vi "Batch_main_with_graph.vi"(1 "Stop":bool=TRUE, 2 "ExpFilePath":path=path "C:/Documents and Settings/Bauerle/Mes documents/takada/HBT6/201612181913.h5") -> ()   [LabVIEW 2013]
uses:
  <vilib>/addons/h5labview2/base/hid_t.ctl
  fpga-bitfile-ref.ctl
  host-subvis/Fast_sequence/sequence slot/slot-use.ctl
  host-subvis/Fast_sequence/sequence slot/triggers.ctl
  host-subvis/Fast_sequence/sequence slot/DAC.ctl
  host-subvis/Fast_sequence/sequence slot/DAC_fastseq-offset.ctl
  host-subvis/Fast_sequence/sequence slot/timing.ctl
  host-subvis/Fast_sequence/sequence slot/jump.ctl
  <vilib>/addons/h5labview2/file/H5Fmode.ctl
  <vilib>/addons/h5labview2/base/lib_path.vi
  <vilib>/addons/h5labview2/base/H5Equery.vi
  <vilib>/FPGAPlugInAG/sbRIO-9602/niLvFpga_Close_sbRIO-9602.vi
  <vilib>/addons/h5labview2/dataset/H5Dread.llb/H5Dread.xnode
  <vilib>/addons/h5labview2/attrib/H5Aread.llb/H5Aread.xnode
  <vilib>/rvi/interface/nirviCloseFPGA/nirviCloseFPGA.xnode
  FPGA Bitfiles/fpga-clean1_FPGATarget_FPGAMAINlock-in_FC21E42C.lvbitx
  <vilib>/addons/h5labview2/attrib/H5Awrite.llb/H5Awrite.xnode
  <vilib>/addons/h5labview2/file/H5F.lvlib
  <vilib>/addons/h5labview2/dataset/H5D.lvlib
  <vilib>/addons/h5labview2/space/H5S.lvlib
panel:
  out "Remaning time (min)":dbl
  in  "temp file interval (ms)":i32=600
  in  "get variable interval (ms)":i32=300
  out "Graph":T1(graph)
  in  "Plot parameters":T2
  out "Temp data":sgl[][](array[numeric])
  out "Initial positions":T3(array[cluster])=[{"Name"="AWG", "kind"=7, "Value"=0.0}, {"Name"="Freq", "kind"=6, "Value"=2759965000.0}, {"Name"="Power", "kind"=6, "Value"=-40.0}, {"Name"="sus", "kind"=4, "Value"=0.29998779296875}, {"Name"="rus", "kind"=4, "Value"=0.29998779296875}, {"Name"="rls", "kind"=4, "Value"=0.29998779296875}, {"Name"="sls", "kind"=4, "Value"=0.059967041015625}, {"Name"="suq", "kind"=4, "Value"=-1.75994873046875}, {"Name"="suu", "kind"=4, "Value"=-0.749969482421875}, {"Name"="sur", "kind"=4, "Value"=-1.199951171875}, {"Name"="suc", "kind"=4, "Value"=-0.449981689453125}, {"Name"="sul", "kind"=4, "Value"=-0.89996337890625}, {"Name"="ruq", "kind"=4, "Value"=-1.699981689453125}, {"Name"="ruu", "kind"=4, "Value"=-0.749969482421875}, {"Name"="rur", "kind"=4, "Value"=-1.25}, {"Name"="ruc", "kind"=4, "Value"=-0.399932861328125}, {"Name"="rul", "kind"=4, "Value"=-0.89996337890625}, {"Name"="rlq", "kind"=4, "Value"=-1.7999267578125}, {"Name"="rlu", "kind"=4, "Value"=-0.89996337890625}, {"Name"="rlr", "kind"=4, "Value"=-1.199951171875}, {"Name"="rlc", "kind"=4, "Value"=-0.5999755859375}, {"Name"="rll", "kind"=4, "Value"=-0.749969482421875}, {"Name"="slq", "kind"=4, "Value"=-1.62506103515625}, {"Name"="slu", "kind"=4, "Value"=-0.89996337890625}, {"Name"="slr", "kind"=4, "Value"=-1.150054931640625}, {"Name"="slc", "kind"=4, "Value"=-0.449981689453125}, {"Name"="sll", "kind"=4, "Value"=-0.749969482421875}, {"Name"="tu", "kind"=4, "Value"=-0.89996337890625}, {"Name"="t", "kind"=4, "Value"=-0.89996337890625}, {"Name"="tl", "kind"=4, "Value"=-0.89996337890625}, {"Name"="4:7", "kind"=4, "Value"=-1.00006103515625}]
  in  "Buf size":i32=300
  out "Var index":u64[](array[numeric])=[0, 49, 0]
  out "start read vals":bool=TRUE
  out "Indexes File":u64[](array[numeric])=[8, 21, 0]
  out "Finish":bool=TRUE
  out "error out":errorcluster
  in  "File update interval (sec)":i32=3000000
  out "DAC_lock-in_info":T4={"Kind"=5, "Strings"=["DAC_Lock-in", "10.0.0.2", "V"], "uint64s"=[0, 1, 0, 0], "Doubles"=[1.0, 0.0, -1.0, -1.0, 50.0, 0.10000000149011612], "DAQmx take out list"=[]}
  out "Fast sequence parameters":T11={"Sequence size"=22, "IP address"="10.0.0.2", "Fast-seq-divider"=6661, "Trigger length"=300, "Sample count"=100, "Send all points?"=FALSE, "Upper limit"=1.0, "Lower limit"=-1.0, "Start ramp at"=0, "fast channels"=[{"dummy?"=FALSE, "panel"=0, "channel"=7}, {"dummy?"=FALSE, "panel"=1, "channel"=0}, {"dummy?"=FALSE, "panel"=0, "channel"=5}, {"dummy?"=FALSE, "panel"=1, "channel"=5}, {"dummy?"=FALSE, "panel"=1, "channel"=6}, {"dummy?"=FALSE, "panel"=1, "channel"=2}, {"dummy?"=FALSE, "panel"=2, "channel"=2}, {"dummy?"=FALSE, "panel"=2, "channel"=3}, {"dummy?"=FALSE, "panel"=2, "channel"=0}, {"dummy?"=FALSE, "panel"=2, "channel"=7}, {"dummy?"=FALSE, "panel"=3, "channel"=0}, {"dummy?"=FALSE, "panel"=2, "channel"=5}, {"dummy?"=FALSE, "panel"=3, "channel"=2}, {"dummy?"=FALSE, "panel"=3, "channel"=3}, {"dummy?"=FALSE, "panel"=3, "channel"=4}, {"dummy?"=FALSE, "panel"=4, "channel"=7}], "fastseq"=[{"use"=enum."triggers", "Triggers"={"triggers"={"1"=TRUE, "2"=TRUE, "3"=FALSE, "4"=FALSE}, "stop"=FALSE}, "DAC"={"FastChanNum"=0, "DAC offset"=0.0}, "timing"=0.0, "slot#"=0}, {"use"=enum."timing", "Triggers"={"triggers"={"1"=FALSE, "2"=FALSE, "3"=FALSE, "4"=FALSE}, "stop"=FALSE}, "DAC"={"FastChanNum"=0, "DAC offset"=0.0}, "timing"=1.0, "slot#"=0}, {"use"=enum."triggers", "Triggers"={"triggers"={"1"=TRUE, "2"=FALSE, "3"=FALSE, "4"=FALSE}, "stop"=FALSE}, "DAC"={"FastChanNum"=0, "DAC offset"=0.0}, "timing"=0.0, "slot#"=0}, {"use"=enum."timing", "Triggers"={"triggers"={"1"=FALSE, "2"=FALSE, "3"=FALSE, "4"=FALSE}, "stop"=FALSE}, "DAC"={"FastChanNum"=0, "DAC offset"=0.0}, "timing"=1.0, "slot#"=0}, {"use"=enum."DAC", "Triggers"={"triggers"={"1"=FALSE, "2"=FALSE, "3"=FALSE, "4"=FALSE}, "stop"=FALSE}, "DAC"={"FastChanNum"=1, "DAC offset"=0.0}, "timing"=0.0, "slot#"=0}, {"use"=enum."DAC", "Triggers"={"triggers"={"1"=FALSE, "2"=FALSE, "3"=FALSE, "4"=FALSE}, "stop"=FALSE}, "DAC"={"FastChanNum"=0, "DAC offset"=0.0}, "timing"=0.0, "slot#"=0}, {"use"=enum."DAC", "Triggers"={"triggers"={"1"=FALSE, "2"=FALSE, "3"=FALSE, "4"=FALSE}, "stop"=FALSE}, "DAC"={"FastChanNum"=4, "DAC offset"=0.0}, "timing"=0.0, "slot#"=0}, {"use"=enum."DAC", "Triggers"={"triggers"={"1"=FALSE, "2"=FALSE, "3"=FALSE, "4"=FALSE}, "stop"=FALSE}, "DAC"={"FastChanNum"=3, "DAC offset"=0.0}, "timing"=0.0, "slot#"=0}, {"use"=enum."DAC", "Triggers"={"triggers"={"1"=FALSE, "2"=FALSE, "3"=FALSE, "4"=FALSE}, "stop"=FALSE}, "DAC"={"FastChanNum"=7, "DAC offset"=0.0}, "timing"=0.0, "slot#"=0}, {"use"=enum."DAC", "Triggers"={"triggers"={"1"=FALSE, "2"=FALSE, "3"=FALSE, "4"=FALSE}, "stop"=FALSE}, "DAC"={"FastChanNum"=6, "DAC offset"=0.0}, "timing"=0.0, "slot#"=0}, {"use"=enum."DAC", "Triggers"={"triggers"={"1"=FALSE, "2"=FALSE, "3"=FALSE, "4"=FALSE}, "stop"=FALSE}, "DAC"={"FastChanNum"=10, "DAC offset"=0.0}, "timing"=0.0, "slot#"=0}, {"use"=enum."DAC", "Triggers"={"triggers"={"1"=FALSE, "2"=FALSE, "3"=FALSE, "4"=FALSE}, "stop"=FALSE}, "DAC"={"FastChanNum"=9, "DAC offset"=0.0}, "timing"=0.0, "slot#"=0}, {"use"=enum."timing", "Triggers"={"triggers"={"1"=FALSE, "2"=FALSE, "3"=FALSE, "4"=FALSE}, "stop"=FALSE}, "DAC"={"FastChanNum"=0, "DAC offset"=0.0}, "timing"=10.0, "slot#"=0}, {"use"=enum."DAC", "Triggers"={"triggers"={"1"=FALSE, "2"=FALSE, "3"=FALSE, "4"=FALSE}, "stop"=FALSE}, "DAC"={"FastChanNum"=1, "DAC offset"=0.0}, "timing"=0.0, "slot#"=0}, {"use"=enum."DAC", "Triggers"={"triggers"={"1"=FALSE, "2"=FALSE, "3"=FALSE, "4"=FALSE}, "stop"=FALSE}, "DAC"={"FastChanNum"=0, "DAC offset"=0.0}, "timing"=0.0, "slot#"=0}, {"use"=enum."DAC", "Triggers"={"triggers"={"1"=FALSE, "2"=FALSE, "3"=FALSE, "4"=FALSE}, "stop"=FALSE}, "DAC"={"FastChanNum"=4, "DAC offset"=0.0}, "timing"=0.0, "slot#"=0}, {"use"=enum."DAC", "Triggers"={"triggers"={"1"=FALSE, "2"=FALSE, "3"=FALSE, "4"=FALSE}, "stop"=FALSE}, "DAC"={"FastChanNum"=3, "DAC offset"=0.0}, "timing"=0.0, "slot#"=0}, {"use"=enum."DAC", "Triggers"={"triggers"={"1"=FALSE, "2"=FALSE, "3"=FALSE, "4"=FALSE}, "stop"=FALSE}, "DAC"={"FastChanNum"=7, "DAC offset"=0.0}, "timing"=0.0, "slot#"=0}, {"use"=enum."DAC", "Triggers"={"triggers"={"1"=FALSE, "2"=FALSE, "3"=FALSE, "4"=FALSE}, "stop"=FALSE}, "DAC"={"FastChanNum"=6, "DAC offset"=0.0}, "timing"=0.0, "slot#"=0}, {"use"=enum."DAC", "Triggers"={"triggers"={"1"=FALSE, "2"=FALSE, "3"=FALSE, "4"=FALSE}, "stop"=FALSE}, "DAC"={"FastChanNum"=10, "DAC offset"=0.0}, "timing"=0.0, "slot#"=0}, {"use"=enum."DAC", "Triggers"={"triggers"={"1"=FALSE, "2"=FALSE, "3"=FALSE, "4"=FALSE}, "stop"=FALSE}, "DAC"={"FastChanNum"=9, "DAC offset"=0.0}, "timing"=0.0, "slot#"=0}, {"use"=enum."jump", "Triggers"={"triggers"={"1"=FALSE, "2"=FALSE, "3"=FALSE, "4"=FALSE}, "stop"=FALSE}, "DAC"={"FastChanNum"=0, "DAC offset"=0.0}, "timing"=0.0, "slot#"=21}]} {"fastseq"."DAC"."DAC offset" min=-1 max=0.5; "fastseq"."DAC"."FastChanNum" max=15 step=1; "fastseq"."slot#" max=4095}
  out "Timings":dbl[][](array[numeric])=[[2417234066.0, 52858.0]] format="%^_3e"
  out "Indexes":i32[](array[numeric])=[8, 21, 0]
  out "sweep_dim":u64[](array[numeric])=[11, 61, 61]
  out "Readout parameters":T12(array[cluster])=[{"Kind"=0, "Strings"=["ADC", "", "V", "sud;rud;rld;sld", "nA;nA;nA;nA", "100.0;100.0;100.0;100.0"], "uint64s"=[5, 4, 250000, 1, 100, 10106, 1000000, 10000, 0, 1], "Doubles"=[1.0], "DAQmx take out list"=["", ""]}]
  out "Exp_params":T15={"filename"="201612181913", "ExpFilePath"=path "C:/Documents and Settings/Bauerle/Mes documents/takada/HBT6/201612181913.h5", "File Ref list"=[16777217, 33554433, 16777216, 33554432], "sweep_dim"=[11, 61, 61], "sweep_list"=["suq", "ruq", "rlq", "slq", "sur", "rur", "rlr", "slr", "suc", "ruc", "rlc", "slc"], "readout_list"=["sud", "rud", "rld", "sld"], "Sweep instrument bools"=[[0, 0], [0, 0], [0, 0], [0, 0], [0, 0], [0, 0], [0, 0], [0, 0], [0, 0], [0, 0], [0, 0], [0, 0], [0, 0], [0, 0], [0, 0], [0, 0], [0, 0], [0, 0], [0, 0], [0, 0], [0, 0], [0, 0], [0, 0], [0, 0], [0, 0], [0, 0], [0, 0], [0, 0], [0, 0], [0, 0], [0, 0], [0, 0], [0, 0], [0, 0], [0, 0], [0, 0], [0, 0], [0, 0], [0, 0], [0, 0], [0, 0]], "Read out instrument bools"=[[1, 0]], "Experimental bool list"=[TRUE, TRUE], "Initial move"=[{"Name"="None", "kind"=100, "Value"=0.0}], "FPGA Ref"=refnum, "Inst_parameters"={"ConfigFilePath"=path "\\\\10.0.0.7\\takada2/DATA/HBT6/data/Configs/conf_20161218_fc_load.h5", "Inst_list"=["ADC", "AWG", "Freq", "Power", "sus", "rus", "rls", "sls", "suq", "suu", "sur", "suc", "sul", "ruq", "ruu", "rur", "ruc", "rul", "rlq", "rlu", "rlr", "rlc", "rll", "slq", "slu", "slr", "slc", "sll", "tu", "t", "tl", "fast_sequence", "4:7", "suc_load", "sur_load", "ruc_load", "rur_load", "rlc_load", "rlr_load", "slc_load", "slr_load", "load_time"], "fast_mode"=[1, 0], "Wait_times"=[1, 1, 1, 1], "Inst_array"=[{"Kind"=0, "Strings"=["ADC", "", "V", "sud;rud;rld;sld", "nA;nA;nA;nA", "100.0;100.0;100.0;100.0"], "uint64s"=[5, 4, 250000, 1, 100, 10106, 1000000, 1, 0, 1], "Doubles"=[1.0], "DAQmx take out list"=[]}, {"Kind"=7, "Strings"=["AWG", "10.0.0.4", "", "C:\\Documents and Settings\\Bauerle\\Mes documents\\Bautze\\FPGA-clean_works_1.13.6_batchtest\\Python\\AWG", "dummy", "SAWnstrig_v4.py"], "uint64s"=[2, 0, 0, 3, 0, 0, 0, 0, 0, 0, 0, 0, 0, 0], "Doubles"=[1200000000.0, 1.0, 0.0, 1.0, 0.0, 1.0, 0.0, 1.0, 0.0, 1.0, 0.0, 1.0, 0.0], "DAQmx take out list"=[]}, {"Kind"=6, "Strings"=["Freq", "0:19", "GHz"], "uint64s"=[1, 0, 0, 0, 2, 0, 0, 0], "Doubles"=[2.0, -30.0, 200.0, 100.0, 0.0, 6.000999927520752, 9.000000318337698e-06, 30.0, -145.0], "DAQmx take out list"=[]}, {"Kind"=6, "Strings"=["Power", "0:19", "GHz"], "uint64s"=[1, 0, 1, 0, 2, 0, 0, 1], "Doubles"=[2.0, -30.0, 200.0, 100.0, 0.0, 6.000999927520752, 9.000000318337698e-06, 30.0, -145.0], "DAQmx take out list"=[]}, {"Kind"=4, "Strings"=["sus", "10.0.0.2", "mV"], "uint64s"=[0, 1], "Doubles"=[1.0, -1.0, 1.0, -1.0, 1.0], "DAQmx take out list"=[]}, {"Kind"=4, "Strings"=["rus", "10.0.0.2", "mV"], "uint64s"=[0, 2], "Doubles"=[1.0, -1.0, 1.0, -1.0, 1.0], "DAQmx take out list"=[]}, {"Kind"=4, "Strings"=["rls", "10.0.0.2", "mV"], "uint64s"=[0, 3], "Doubles"=[1.0, -1.0, 1.0, -1.0, 1.0], "DAQmx take out list"=[]}, {"Kind"=4, "Strings"=["sls", "10.0.0.2", "mV"], "uint64s"=[0, 4], "Doubles"=[1.0, -1.0, 1.0, -1.0, 1.0], "DAQmx take out list"=[]}, {"Kind"=4, "Strings"=["suq", "10.0.0.2", "V"], "uint64s"=[0, 5], "Doubles"=[0.30000001192092896, -2.0, 1.0, -1.0, 1.0], "DAQmx take out list"=[]}, {"Kind"=4, "Strings"=["suu", "10.0.0.2", "V"], "uint64s"=[0, 6], "Doubles"=[0.30000001192092896, -2.0, 1.0, -1.0, 1.0], "DAQmx take out list"=[]}, {"Kind"=4, "Strings"=["sur", "10.0.0.2", "V"], "uint64s"=[0, 7], "Doubles"=[0.30000001192092896, -2.0, 1.0, -1.0, 1.0], "DAQmx take out list"=[]}, {"Kind"=4, "Strings"=["suc", "10.0.0.2", "V"], "uint64s"=[1, 0], "Doubles"=[0.30000001192092896, -2.0, 1.0, -1.0, 1.0], "DAQmx take out list"=[]}, {"Kind"=4, "Strings"=["sul", "10.0.0.2", "V"], "uint64s"=[1, 1], "Doubles"=[0.30000001192092896, -2.0, 1.0, -1.0, 1.0], "DAQmx take out list"=[]}, {"Kind"=4, "Strings"=["ruq", "10.0.0.2", "V"], "uint64s"=[1, 2], "Doubles"=[0.30000001192092896, -2.0, 1.0, -1.0, 1.0], "DAQmx take out list"=[]}, {"Kind"=4, "Strings"=["ruu", "10.0.0.2", "V"], "uint64s"=[1, 3], "Doubles"=[0.30000001192092896, -2.0, 1.0, -1.0, 1.0], "DAQmx take out list"=[]}, {"Kind"=4, "Strings"=["rur", "10.0.0.2", "V"], "uint64s"=[1, 5], "Doubles"=[0.30000001192092896, -2.0, 1.0, -1.0, 1.0], "DAQmx take out list"=[]}, {"Kind"=4, "Strings"=["ruc", "10.0.0.2", "V"], "uint64s"=[1, 6], "Doubles"=[0.30000001192092896, -2.0, 1.0, -1.0, 1.0], "DAQmx take out list"=[]}, {"Kind"=4, "Strings"=["rul", "10.0.0.2", "V"], "uint64s"=[1, 7], "Doubles"=[0.30000001192092896, -2.0, 1.0, -1.0, 1.0], "DAQmx take out list"=[]}, {"Kind"=4, "Strings"=["rlq", "10.0.0.2", "V"], "uint64s"=[2, 0], "Doubles"=[0.30000001192092896, -2.0, 1.0, -1.0, 1.0], "DAQmx take out list"=[]}, {"Kind"=4, "Strings"=["rlu", "10.0.0.2", "V"], "uint64s"=[2, 1], "Doubles"=[0.30000001192092896, -2.0, 1.0, -1.0, 1.0], "DAQmx take out list"=[]}, {"Kind"=4, "Strings"=["rlr", "10.0.0.2", "V"], "uint64s"=[2, 2], "Doubles"=[0.30000001192092896, -2.0, 1.0, -1.0, 1.0], "DAQmx take out list"=[]}, {"Kind"=4, "Strings"=["rlc", "10.0.0.2", "V"], "uint64s"=[2, 3], "Doubles"=[0.30000001192092896, -2.0, 1.0, -1.0, 1.0], "DAQmx take out list"=[]}, {"Kind"=4, "Strings"=["rll", "10.0.0.2", "V"], "uint64s"=[2, 4], "Doubles"=[0.30000001192092896, -2.0, 1.0, -1.0, 1.0], "DAQmx take out list"=[]}, {"Kind"=4, "Strings"=["slq", "10.0.0.2", "V"], "uint64s"=[2, 5], "Doubles"=[0.30000001192092896, -2.0, 1.0, -1.0, 1.0], "DAQmx take out list"=[]}, {"Kind"=4, "Strings"=["slu", "10.0.0.2", "V"], "uint64s"=[2, 6], "Doubles"=[0.30000001192092896, -2.0, 1.0, -1.0, 1.0], "DAQmx take out list"=[]}, {"Kind"=4, "Strings"=["slr", "10.0.0.2", "V"], "uint64s"=[2, 7], "Doubles"=[0.30000001192092896, -2.0, 1.0, -1.0, 1.0], "DAQmx take out list"=[]}, {"Kind"=4, "Strings"=["slc", "10.0.0.2", "V"], "uint64s"=[3, 0], "Doubles"=[0.30000001192092896, -2.0, 1.0, -1.0, 1.0], "DAQmx take out list"=[]}, {"Kind"=4, "Strings"=["sll", "10.0.0.2", "V"], "uint64s"=[3, 1], "Doubles"=[0.30000001192092896, -2.0, 1.0, -1.0, 1.0], "DAQmx take out list"=[]}, {"Kind"=4, "Strings"=["tu", "10.0.0.2", "V"], "uint64s"=[3, 2], "Doubles"=[0.30000001192092896, -2.0, 1.0, -1.0, 1.0], "DAQmx take out list"=[]}, {"Kind"=4, "Strings"=["t", "10.0.0.2", "V"], "uint64s"=[3, 3], "Doubles"=[0.30000001192092896, -2.0, 1.0, -1.0, 1.0], "DAQmx take out list"=[]}, {"Kind"=4, "Strings"=["tl", "10.0.0.2", "V"], "uint64s"=[3, 4], "Doubles"=[0.30000001192092896, -2.0, 1.0, -1.0, 1.0], "DAQmx take out list"=[]}, {"Kind"=9, "Strings"=["fast_sequence", "10.0.0.2", "V"], "uint64s"=[6661, 300, 100, 0, 7, 8, 5, 13, 14, 10, 18, 19, 16, 23, 24, 21, 26, 27, 28, 39, 0], "Doubles"=[1.0, -1.0, -1.0, -1.0], "DAQmx take out list"=[]}, {"Kind"=4, "Strings"=["4:7", "10.0.0.2", "V"], "uint64s"=[4, 7], "Doubles"=[0.30000001192092896, -2.0, 1.0, -1.0, 1.0], "DAQmx take out list"=[]}, {"Kind"=10, "Strings"=["suc_load", "10.0.0.2", "V"], "uint64s"=[4, 0], "Doubles"=[0.5, -0.5], "DAQmx take out list"=[]}, {"Kind"=10, "Strings"=["sur_load", "10.0.0.2", "V"], "uint64s"=[5, 0], "Doubles"=[0.5, -0.5], "DAQmx take out list"=[]}, {"Kind"=10, "Strings"=["ruc_load", "10.0.0.2", "V"], "uint64s"=[6, 0], "Doubles"=[0.5, -0.5], "DAQmx take out list"=[]}, {"Kind"=10, "Strings"=["rur_load", "10.0.0.2", "V"], "uint64s"=[7, 0], "Doubles"=[0.5, -0.5], "DAQmx take out list"=[]}, {"Kind"=10, "Strings"=["rlc_load", "10.0.0.2", "V"], "uint64s"=[8, 0], "Doubles"=[0.5, -0.5], "DAQmx take out list"=[]}, {"Kind"=10, "Strings"=["rlr_load", "10.0.0.2", "V"], "uint64s"=[9, 0], "Doubles"=[0.5, -0.5], "DAQmx take out list"=[]}, {"Kind"=10, "Strings"=["slc_load", "10.0.0.2", "V"], "uint64s"=[10, 0], "Doubles"=[0.5, -0.5], "DAQmx take out list"=[]}, {"Kind"=10, "Strings"=["slr_load", "10.0.0.2", "V"], "uint64s"=[11, 0], "Doubles"=[0.5, -0.5], "DAQmx take out list"=[]}, {"Kind"=10, "Strings"=["load_time", "10.0.0.2", "ms"], "uint64s"=[12, 0], "Doubles"=[1000.0, -0.009999999776482582], "DAQmx take out list"=[]}]}} {"File Ref list" format="%.0x"}
  out "Sweep inst info":T12(array[cluster])=[{"Kind"=4, "Strings"=["suq", "10.0.0.2", "V"], "uint64s"=[0, 5], "Doubles"=[0.30000001192092896, -2.0, 1.0, -1.0, 1.0], "DAQmx take out list"=[]}, {"Kind"=4, "Strings"=["ruq", "10.0.0.2", "V"], "uint64s"=[1, 2], "Doubles"=[0.30000001192092896, -2.0, 1.0, -1.0, 1.0], "DAQmx take out list"=[]}, {"Kind"=4, "Strings"=["rlq", "10.0.0.2", "V"], "uint64s"=[2, 0], "Doubles"=[0.30000001192092896, -2.0, 1.0, -1.0, 1.0], "DAQmx take out list"=[]}, {"Kind"=4, "Strings"=["slq", "10.0.0.2", "V"], "uint64s"=[2, 5], "Doubles"=[0.30000001192092896, -2.0, 1.0, -1.0, 1.0], "DAQmx take out list"=[]}, {"Kind"=4, "Strings"=["sur", "10.0.0.2", "V"], "uint64s"=[0, 7], "Doubles"=[0.30000001192092896, -2.0, 1.0, -1.0, 1.0], "DAQmx take out list"=[]}, {"Kind"=4, "Strings"=["rur", "10.0.0.2", "V"], "uint64s"=[1, 5], "Doubles"=[0.30000001192092896, -2.0, 1.0, -1.0, 1.0], "DAQmx take out list"=[]}, {"Kind"=4, "Strings"=["rlr", "10.0.0.2", "V"], "uint64s"=[2, 2], "Doubles"=[0.30000001192092896, -2.0, 1.0, -1.0, 1.0], "DAQmx take out list"=[]}, {"Kind"=4, "Strings"=["slr", "10.0.0.2", "V"], "uint64s"=[2, 7], "Doubles"=[0.30000001192092896, -2.0, 1.0, -1.0, 1.0], "DAQmx take out list"=[]}, {"Kind"=4, "Strings"=["suc", "10.0.0.2", "V"], "uint64s"=[1, 0], "Doubles"=[0.30000001192092896, -2.0, 1.0, -1.0, 1.0], "DAQmx take out list"=[]}, {"Kind"=4, "Strings"=["ruc", "10.0.0.2", "V"], "uint64s"=[1, 6], "Doubles"=[0.30000001192092896, -2.0, 1.0, -1.0, 1.0], "DAQmx take out list"=[]}, {"Kind"=4, "Strings"=["rlc", "10.0.0.2", "V"], "uint64s"=[2, 3], "Doubles"=[0.30000001192092896, -2.0, 1.0, -1.0, 1.0], "DAQmx take out list"=[]}, {"Kind"=4, "Strings"=["slc", "10.0.0.2", "V"], "uint64s"=[3, 0], "Doubles"=[0.30000001192092896, -2.0, 1.0, -1.0, 1.0], "DAQmx take out list"=[]}]
  # "total"
  # "nb of calls"
  # "average"
  # "total time"
  # "read config"
  # "plot loop"
  # "save data"
  # "config instr"
  # "FPGA init"
  # "voltmeter init"
  # "initial move"
  # "read init values"
  # "meas loop"
  # "move + wait"
  # "FPGA config"
  # "FPGA start"
  # "FPGA stop"
  # "read data"
  # "clear buffer"
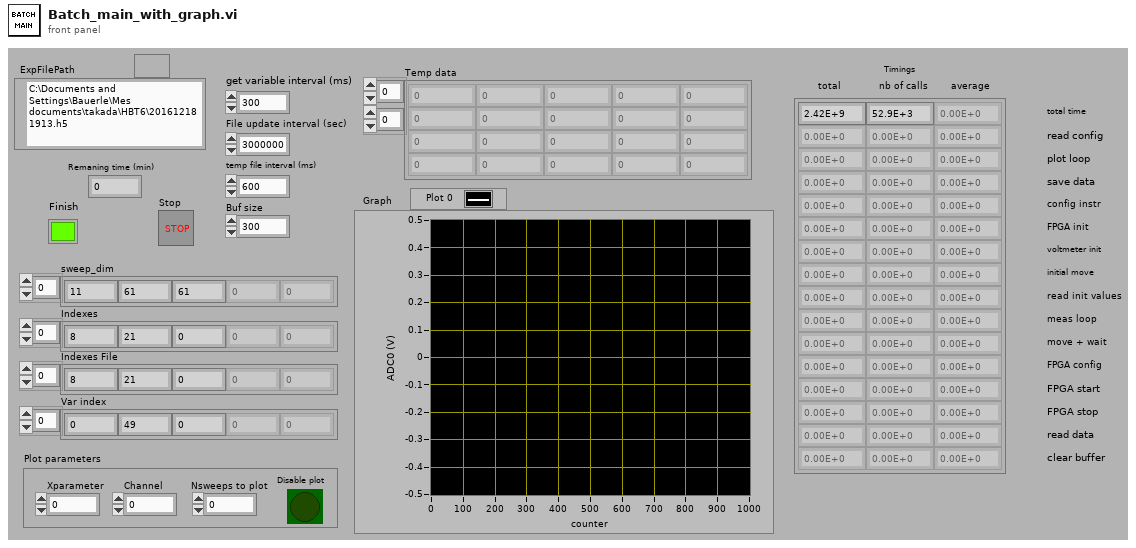
[diagram p1: front panel]
types:
  T1 = cluster{"Sweep buffer":dbl[], "Readout buffer":dbl[]}
  T2 = cluster{"Disable plot":bool, "Nsweeps to plot":dbl, "Channel":dbl, "Xparameter":dbl, "Readout buffer":dbl[][], "Sweep buffer":dbl[][]}
  T3 = cluster{"Name":string, "kind":u64, "Value":dbl}[]
  T4 = cluster{"Kind":u16, "Strings":string[], "uint64s":u64[], "Doubles":dbl[], "DAQmx take out list":refnum<k21>[]}
  T5 = typedef "slot-use.ctl" = enum8{"DAC", "timing", "triggers", "jump"}
  T6 = typedef "triggers.ctl" = cluster{"triggers":cluster{"1":bool, "2":bool, "3":bool, "4":bool}, "stop":bool}
  T7 = typedef "DAC.ctl" = cluster{"FastChanNum":u8, "DAC offset":T8}
  T8 = typedef "DAC_fastseq-offset.ctl" = sgl
  T9 = typedef "timing.ctl" = sgl
  T10 = typedef "jump.ctl" = u16
  T11 = cluster{"Sequence size":u64, "IP address":string, "Fast-seq-divider":u64, "Trigger length":u64, "Sample count":u64, "Send all points?":bool, "Upper limit":dbl, "Lower limit":dbl, "Start ramp at":u64, "fast channels":cluster{"dummy?":bool, "panel":u8, "channel":u8}[], "fastseq":cluster{"use":T5, "Triggers":T6, "DAC":T7, "timing":T9, "slot#":T10}[]}
  T12 = cluster{"Kind":u16, "Strings":string[], "uint64s":u64[], "Doubles":dbl[], "DAQmx take out list":refnum<k21>[]}[]
  T13 = typedef "hid_t.ctl" = i32
  T14 = typedef "fpga-bitfile-ref.ctl" = refnum<k20>
  T15 = cluster{"filename":string, "ExpFilePath":path, "File Ref list":T13[], "sweep_dim":u64[], "sweep_list":string[], "readout_list":string[], "Sweep instrument bools":u64[][], "Read out instrument bools":u64[][], "Experimental bool list":bool[], "Initial move":cluster{"Name":string, "kind":u64, "Value":dbl}[], "FPGA Ref":T14, "Inst_parameters":cluster{"ConfigFilePath":path, "Inst_list":string[], "fast_mode":u8[], "Wait_times":u64[], "Inst_array":cluster{"Kind":u16, "Strings":string[], "uint64s":u64[], "Doubles":dbl[], "DAQmx take out list":refnum<k21>[]}[]}}
  T16 = cluster{"filename":string, "ExpFilePath":path, "File Ref list":T13[], "sweep_dim":u64[], "sweep_list":string[], "readout_list":string[], "Sweep instrument bools":u64[][], "Read out instrument bools":u64[][], "Experimental bool list":bool[], "Initial moves":cluster{"name":string, "parameter":u64, "value":dbl}[], "FPGA Ref":T14, "Inst_parameters":cluster{"ConfigFilePath":path, "Inst_list":string[], "fast_mode":u8[], "Wait_times":u64[], "Inst_array":cluster{"Kind":u16, "Strings":string[], "uint64s":u64[], "Doubles":dbl[], "DAQmx take out list":refnum<k21>[]}[]}}
  T17 = typedef "H5F.lvlib/H5Fmode.ctl" = enum16{"read-only", "read-write", "overwrite", "create new", "open or create"}
  T18 = enum16{"stop", "set divider", "unset ramp mode", "unset stop count", "set pulse lenght", "set ramp", "start"}
  T19 = cluster{"Kind":u16, "Strings":string[], "uint64s":u64[], "Doubles":dbl[], refnum<k21>[]}[]
  T20 = cluster{"use":T5, "Triggers":T6, "DAC":T7, "timing":T9, "slot#":T10}[]
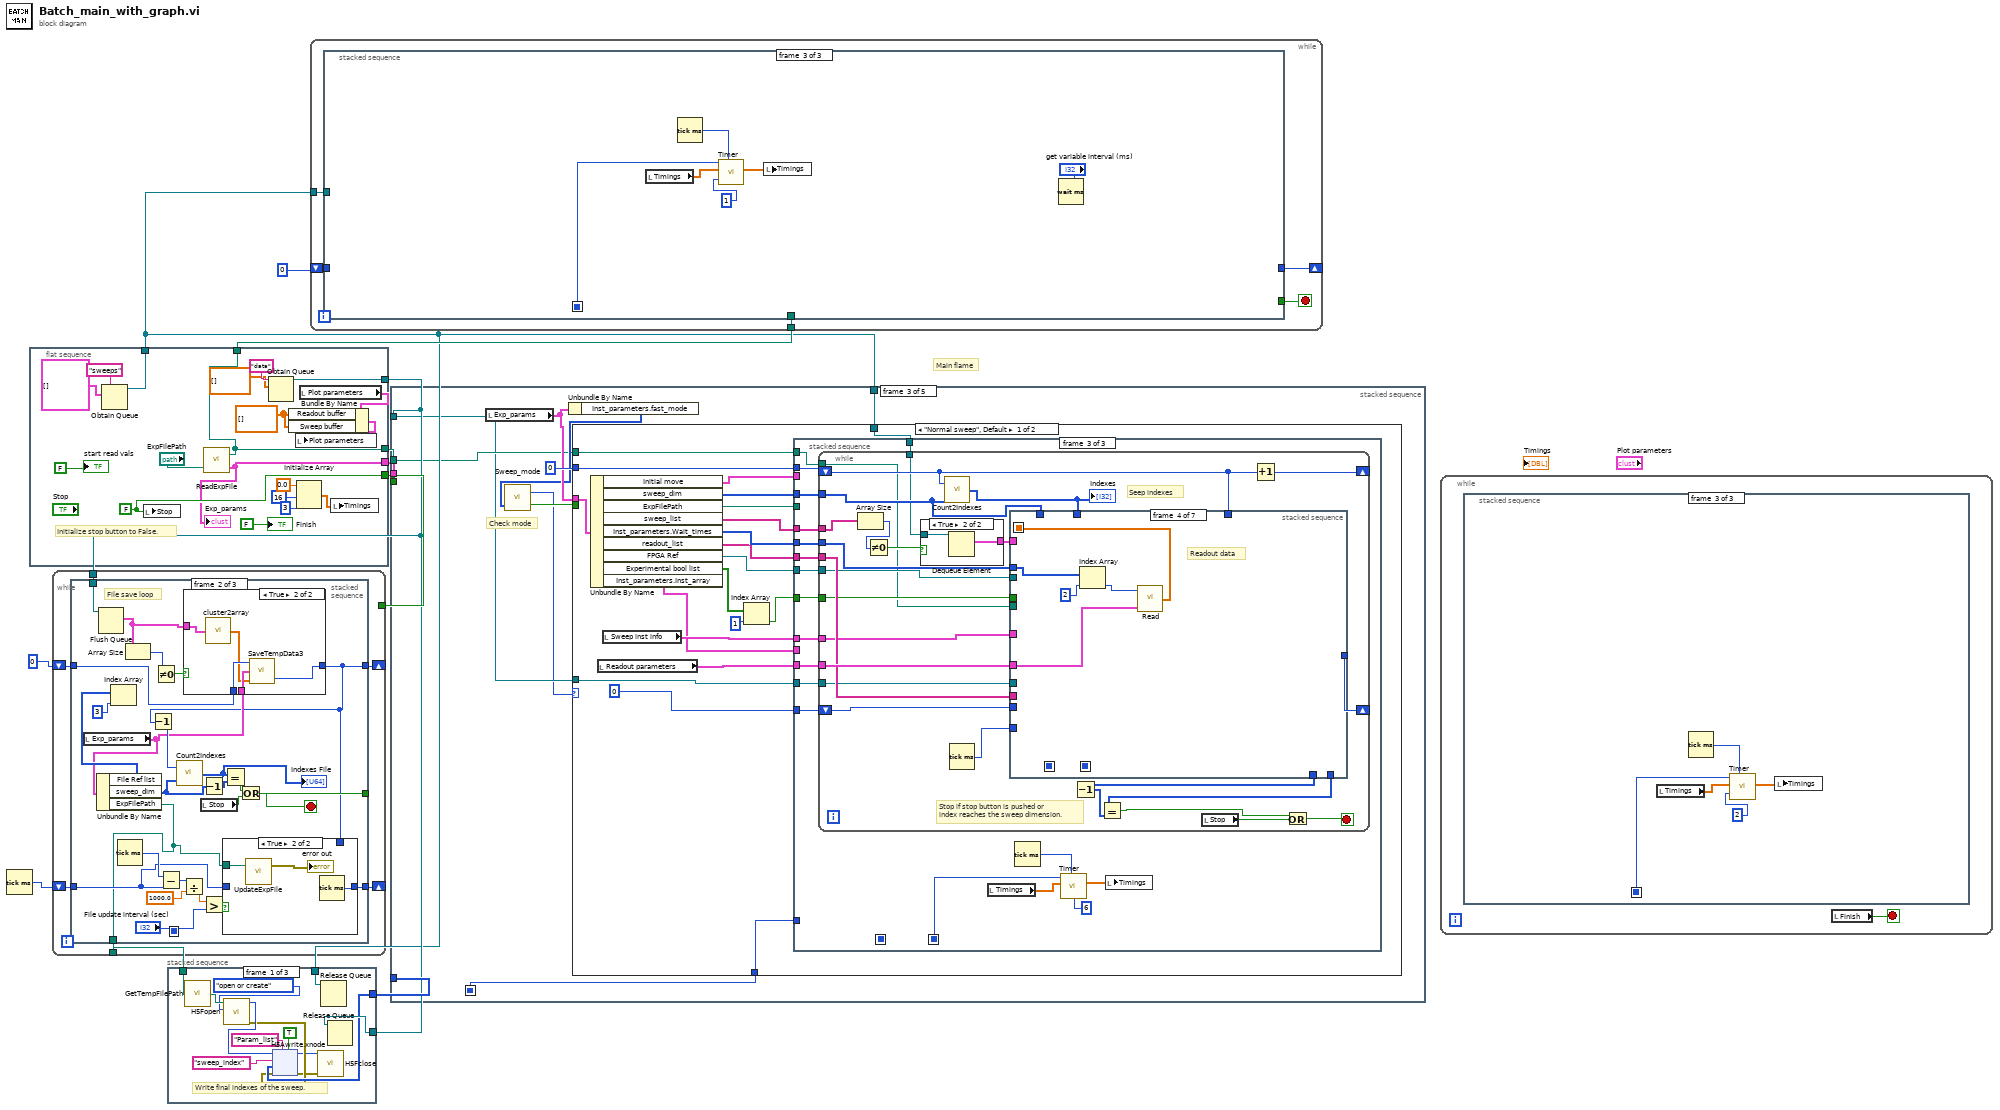
[diagram p0: block diagram]
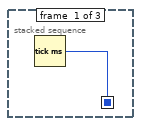
[diagram p2: hidden frame]
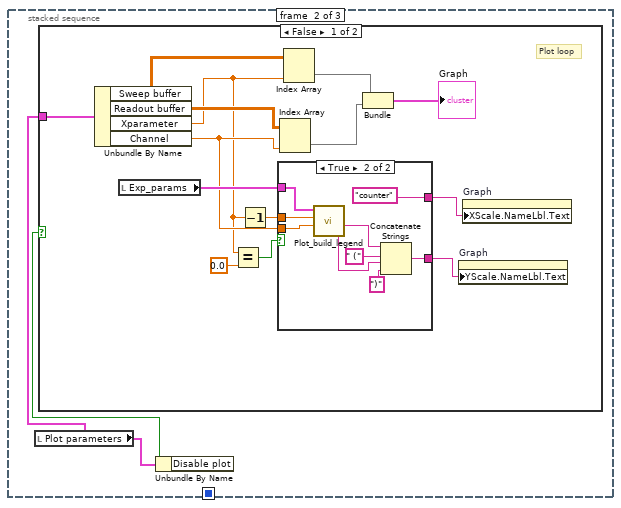
[diagram p3: hidden frame]
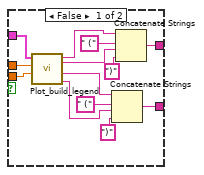
[diagram p4: hidden frame]
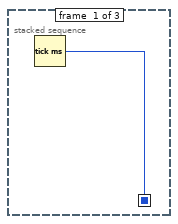
[diagram p6: hidden frame]
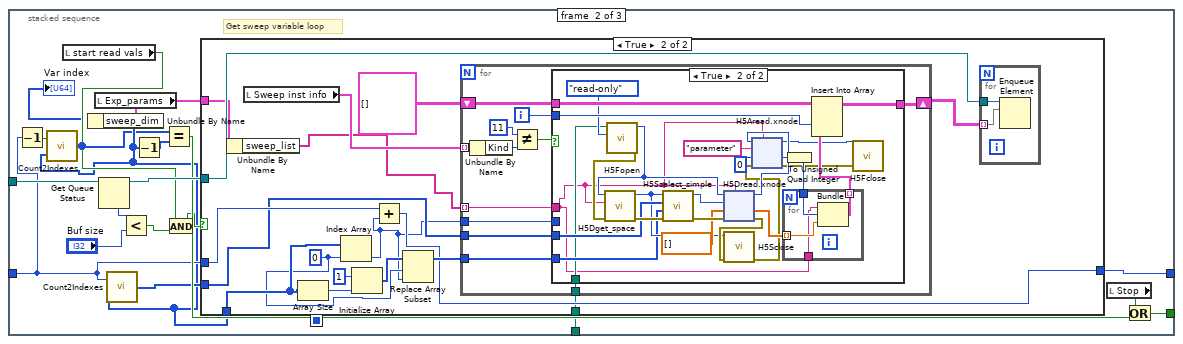
[diagram p7: hidden frame]
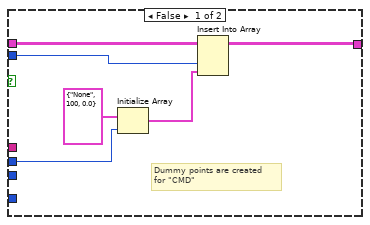
[diagram p9: hidden frame]
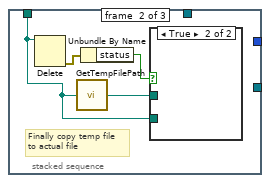
[diagram p10: hidden frame]
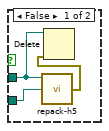
[diagram p11: hidden frame]
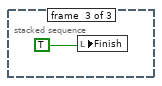
[diagram p12: hidden frame]
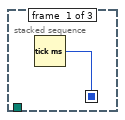
[diagram p13: hidden frame]
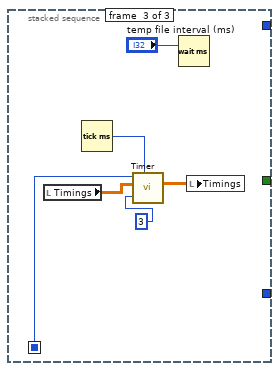
[diagram p16: hidden frame]
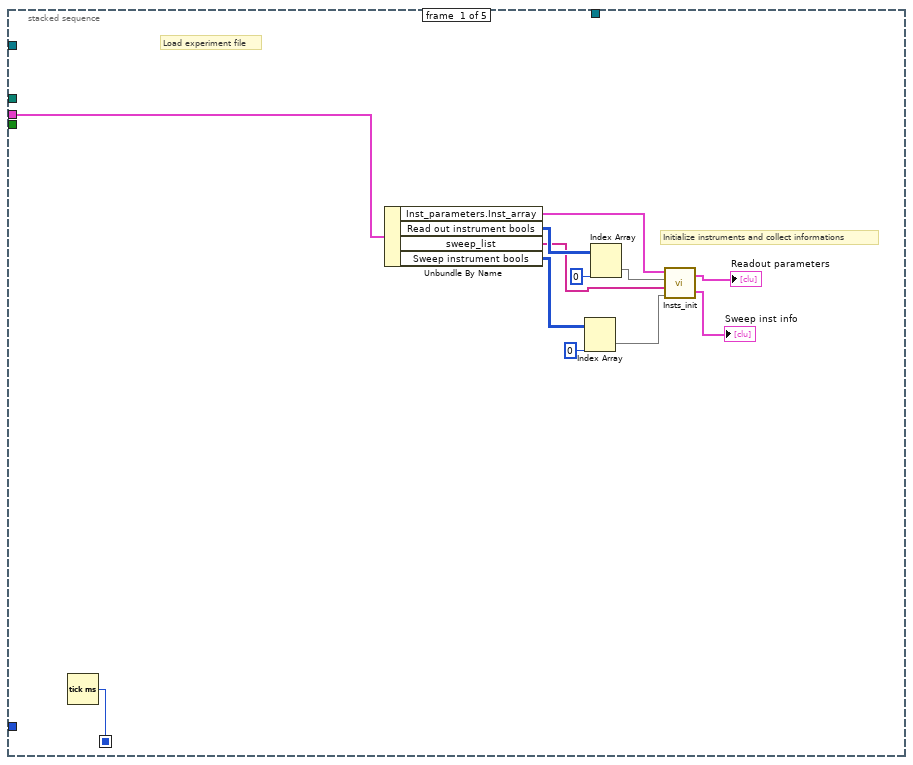
[diagram p17: hidden frame]
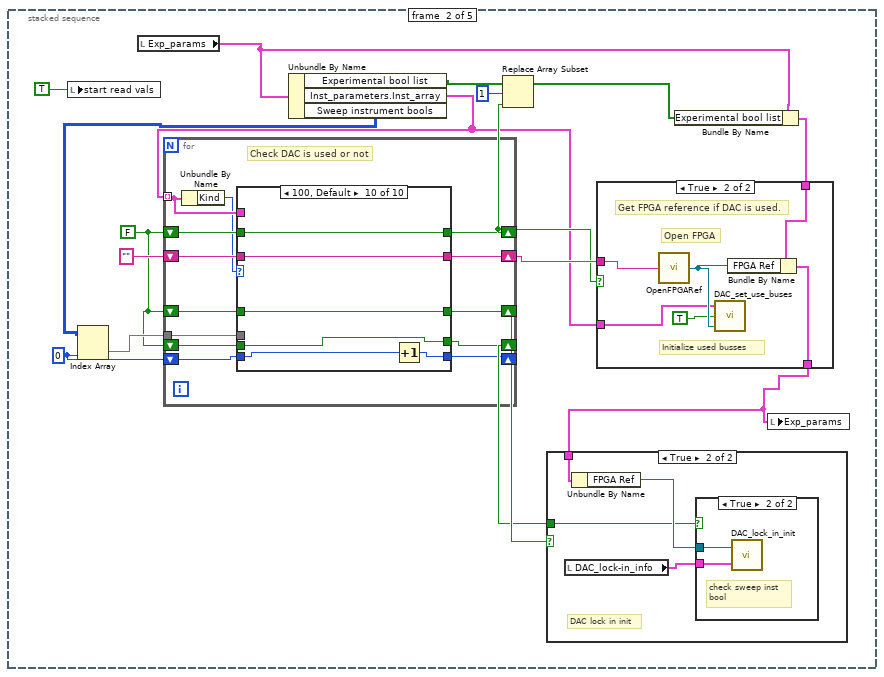
[diagram p18: hidden frame]
diagram:
  # "Main flame"
  n1 = Tick Count (ms)() -> (millisecond timer value=w10:u32)
  n2 = flat-sequence {
    tunnel: [w30] -> w7
    tunnel: [w21] -> w2
    tunnel: [w25] -> w1
    tunnel: [w22] -> w5
    tunnel: [w18] -> w4
    tunnel: [w18] -> w3
    frame #0 {
      w19 = dbl[][] []
      w30 = FALSE
      # "Initialize stop button to False."
      n3 = Obtain Queue(name (unnamed)="sweeps", element data type=cluster{string, "data":u64, dbl}[] []) -> (queue out=w25:refnum<queue>)  [unwired: 3 in, 2 out]
      n4 = local write "Stop"(w30) -> ()
      n5 = call "ReadExpFile.vi"("ExpFilePath"="ExpFilePath") -> ("Exp_params"=w22:T16, "WorkFilePath"=w18:path)  [unwired: 1 in]
      "Exp_params" <- w22
      n6 = Obtain Queue(name (unnamed)="data", element data type=dbl[][] []) -> (queue out=w21:refnum<queue>)  [unwired: 3 in, 2 out]
      n7 = Initialize Array(0.0, 16, 3) -> (w14:dbl[][])
      n8 = local read "Plot parameters"() -> (w16:T2)
      n9 = Bundle By Name(cluster=w16, "Readout buffer"=w19, "Sweep buffer"=w19) -> (w17:T2)
      n10 = local write "Plot parameters"(w17) -> ()
      n11 = local write "Timings"(w14) -> ()
      "Finish" <- FALSE
      "start read vals" <- FALSE
    }
  }
  n12 = while {
    shift-right: [w31] -> _
    shift-left: 0 -> [w36]
    shift-right: [w34] -> _
    shift-left: w10 -> [w35]
    tunnel: [w32] -> w8
    tunnel: w7 -> [_]
    tunnel: w2 -> [w33]
    stop <- w37 stop-if-true
    n13 = stacked-sequence {
      seq-local: [w38 _ _] -> [_ _ w78]
      tunnel: [_ w59 _] -> w37
      tunnel: w36 -> [_ w57 _]
      tunnel: w35 -> [_ w48 _]
      tunnel: [_ w47 _] -> w34
      tunnel: w33 -> [_ w41 _]
      tunnel: [_ w40 _] -> w32
      tunnel: [_ w39 _] -> w31
      frame #0 {
        n14 = Tick Count (ms)() -> (millisecond timer value=w38:u32)
      }
      frame #1 {
        # "File save loop"
        n15 = local read "Exp_params"() -> (w44:T15)
        n16 = Unbundle By Name(w44) -> ("File Ref list"=w45:T13[], "sweep_dim"=w60:u64[], "ExpFilePath"=w40:path)
        n17 = Flush Queue(queue=w41) -> (remaining elements=w42:cluster{dbl[][]}[])  [unwired: 1 in, 2 out]
        n18 = Index Array(array=w45, index=3) -> ()  [unwired: 1 out]
        n19 = Tick Count (ms)() -> (millisecond timer value=w55:u32)
        n20 = Array Size(array=w42) -> (size(s)=w43:i32)
        n21 = Not Equal To 0?(x=w43) -> (x != 0?=w58:bool)
        n22 = Subtract(x=w55, y=w48) -> (x-y=w54:u32)
        n23 = Divide(x=w54, y=1000.0) -> (x/y=w52:dbl)
        n24 = case shown="True" w58 {
          tunnel: w57 -> [w68 w73]
          tunnel: [w68 w72] -> w39
          tunnel: w44 -> [_ w71]
          tunnel: w42 -> [_ w70]
          frame False {
          }
          frame True {
            n25 = call "cluster2array.vi"("temp data"=w70) -> ("temp data array"=w69:dbl[][][])
            n26 = call "SaveTempData3.vi"("temp data"=w69, "Exp_params"=w71, "count"=w73) -> ("count out"=w72:i32)  [unwired: 1 in]
          }
        }
        n27 = Decrement(x=w39) -> (x-1=w56:i32)
        n28 = call "Count2Indexes.vi"("sweep_dim"=w60, "Count"=w56) -> ("Indexes"=w49:u64[])
        "Indexes File" <- w49
        n29 = local read "Stop"() -> (w63:bool)
        n30 = Decrement(x=w60) -> (x-1=w61:u64[])
        n31 = Greater?(x=w52, y="File update interval (sec)") -> (0:w50:bool)
        n32 = Equal?(x=w49, y=w61) -> (x = y?=w62:bool)
        n33 = case shown="True" w50 {
          tunnel: w48 -> [w64 _]
          tunnel: [w64 w66] -> w47
          tunnel: w40 -> [_ w65]
          tunnel: w39 -> [_ _]
          frame False {
          }
          frame True {
            n34 = call "UpdateExpFile.vi"("ExpFilePath"=w65) -> ("error out"=→"error out":errorcluster)  [unwired: 2 in]
            n35 = Tick Count (ms)() -> (millisecond timer value=w66:u32)
          }
        }
        n36 = Or(x=w62, y=w63) -> (x .or. y?=w59:bool)
      }
      frame #2 {
        n37 = local read "Timings"() -> (w74:dbl[][])
        n38 = Tick Count (ms)() -> (millisecond timer value=w77:u32)
        n39 = call "Timer.vi"("index"=3, "Timings in"=w74, "t1"=w78, "t2"=w77) -> ("Timings out"=w75:dbl[][])  [unwired: 2 in]
        n40 = Wait (ms)(milliseconds to wait="temp file interval (ms)") -> ()  [unwired: 1 out]
        n41 = local write "Timings"(w75) -> ()
      }
    }
  }
  n42 = while {
    tunnel: w1 -> [w84]
    shift-right: [w83] -> _
    shift-left: u64 0 -> [w81]
    tunnel: w4 -> [w80]
    stop <- w82 stop-if-true
    n43 = stacked-sequence {
      seq-local: [w85 _ _] -> [_ _ w207]
      tunnel: w84 -> [_ w104 _]
      tunnel: [_ w101 _] -> w83
      tunnel: [_ w98 _] -> w82
      tunnel: w81 -> [_ w90 _]
      tunnel: w80 -> [_ w86 _]
      frame #0 {
        n44 = Tick Count (ms)() -> (millisecond timer value=w85:u32)
      }
      frame #1 {
        # "Get sweep variable loop"
        n45 = Decrement(x=w90) -> (x-1=w91:u64)
        n46 = local read "start read vals"() -> (w92:bool)
        n47 = local read "Exp_params"() -> (w95:T15)
        n48 = Unbundle By Name(w95) -> ("sweep_dim"=w88:u64[])
        n49 = call "Count2Indexes.vi"("sweep_dim"=w88, "Count"=w91) -> ("Indexes"=w87:u64[])
        "Var index" <- w87
        n50 = Get Queue Status(queue=w104) -> (queue out=w100:refnum<queue>, # elements in queue=w103:i32)  [unwired: 2 in, 6 out]
        n51 = call "Count2Indexes.vi"("sweep_dim"=w88, "Count"=w90) -> ("Indexes"=w89:u64[])
        n52 = Less?(x=w103, y="Buf size") -> (x < y?=w93:bool)
        n53 = Decrement(x=w88) -> (x-1=w97:u64[])
        n54 = Equal?(x=w87, y=w97) -> (x = y?=w96:bool)
        n55 = And(x=w92, y=w93) -> (x .and. y?=w94:bool)
        n56 = case shown="True" w94 {
          tunnel: w88 -> [_ w118]
          tunnel: w90 -> [w105 w116]
          tunnel: [w105 w111] -> w101
          tunnel: w100 -> [_ w113]
          tunnel: w89 -> [_ w112]
          tunnel: w95 -> [_ w109]
          tunnel: w86 -> [_ w106]
          frame False {
          }
          frame True {
            w117 = 0
            n57 = Unbundle By Name(w109) -> ("sweep_list"=w108:string[])
            n58 = local read "Sweep inst info"() -> (w110:T12)
            n59 = Array Size(array=w118) -> (size(s)=w121:i32)
            n60 = Index Array(array=w118, index=w117) -> (element=w107:u64)
            n61 = Initialize Array(u32 1, w121) -> (w120:u32[])
            n62 = Add(x=w116, y=w107) -> (x+y=w111:u64)
            n63 = Replace Array Subset(array=w120, new element=w107, index=w117) -> (w115:u32[])
            n64 = for {
              shift-right: [w129] -> w114
              shift-left: cluster{string, "data":u16, dbl}[][] [] -> [w130]
              tunnel: w108 -> [w125] mode=indexing
              tunnel: w115 -> [w131]
              tunnel: w112 -> [w132]
              tunnel: w110 -> [w136] mode=indexing
              tunnel: w107 -> [w128]
              tunnel: w106 -> [w126]
              i -> [w127]
              n65 = Unbundle By Name(w136) -> ("Kind"=w135:u16)
              n66 = Not Equal?(x=11, y=w135) -> (x != y?=w133:bool)
              n67 = case shown="True" w133 {
                tunnel: w132 -> [_ w164]
                tunnel: w131 -> [_ w161]
                tunnel: w125 -> [_ w143]
                tunnel: w130 -> [w142 w155]
                tunnel: [w141 w154] -> w129
                tunnel: w128 -> [w139 _]
                tunnel: w127 -> [w137 w151]
                tunnel: w126 -> [_ w149]
                frame False {
                  # "Dummy points are created\nfor \"CMD\""
                  n68 = Initialize Array(cluster{string, "data":u64, dbl} {"None", "data"=100, 0.0}, w139) -> (w138:cluster{string, "data":u64, dbl}[])
                  n69 = Insert Into Array(array=w142, index (col)=w137, new element=w138) -> (w141:cluster{string, "data":u16, dbl}[][])  [unwired: 1 in]
                }
                frame True {
                  n70 = call <vilib>:"H5Fopen.vi"("mode (read-only)"=H5Fmode."read-only" ("mode"), "path"=w149) -> ("error out"=w144:errorcluster, "ref out"=w148:T13)  [unwired: 8 in]
                  n71 = call <vilib>:"H5Dget_space.vi"("error in (no error)"=w144, "obj (.)"=w143, "ref in"=w148) -> ("error out"=w168:errorcluster, "space out"=w162:T13)  [unwired: 7 in]
                  n72 = call <vilib>:"H5Sselect_simple.vi"("error in (no error)"=w168, "count"=w161, "start"=w164, "space in"=w162) -> ("error out"=w167:errorcluster, "space out"=w163:T13)  [unwired: 6 in]
                  n73 = xnode "H5Dread.xnode"("dataset name (this)"=w143, "error in (no error)"=w167, "default"=dbl[] [], "file space"=w163, "ref in"=w148) -> ("error out"=w166:errorcluster, "data"=w160:dbl[], "ref out"=w157:T13)  [unwired: 1 in, 1 out]
                  n74 = call <vilib>:"H5Sclose.vi"("error in (no error)"=w166, "space in"=w162) -> ("error out"=w147:errorcluster)  [unwired: 9 in]
                  n75 = xnode "H5Aread.xnode"("object name"=w143, "error in (no error)"=w147, "default"=u16 0, "attrib name"="parameter", "ref in"=w157) -> ("error out"=w146:errorcluster, "data"=w156:u16, "ref out"=w145:T13)  [unwired: 1 in, 1 out]
                  n76 = To Unsigned Quad Integer(1:w156) -> (0:w152:u64)
                  n77 = for {
                    tunnel: w160 -> [w187] mode=indexing
                    tunnel: w152 -> [w186]
                    tunnel: [w185] -> w153 mode=indexing
                    tunnel: w143 -> [w184]
                    n78 = Bundle(w184, w186, w187) -> (w185:cluster{string, u64, dbl})  [unwired: 1 in]
                  }
                  n79 = Insert Into Array(array=w155, index (col)=w151, new element=w153) -> (w154:cluster{string, "data":u16, dbl}[][])  [unwired: 1 in]
                  n80 = call <vilib>:"H5Fclose.vi"("error in (no error)"=w146, "ref"=w145) -> ()  [unwired: 9 in, 1 out]
                }
              }
            }
            n81 = for {
              tunnel: w114 -> [w124] mode=indexing
              tunnel: w113 -> [w123]
              n82 = Enqueue Element(queue=w123, element=w124) -> ()  [unwired: 2 in, 3 out]
            }
          }
        }
        n83 = local read "Stop"() -> (w99:bool)
        n84 = Or(x=w99, y=w96) -> (x .or. y?=w98:bool)
      }
      frame #2 {
        n85 = local read "Timings"() -> (w203:dbl[][])
        n86 = Tick Count (ms)() -> (millisecond timer value=w206:u32)
        n87 = call "Timer.vi"("index"=1, "Timings in"=w203, "t1"=w207, "t2"=w206) -> ("Timings out"=w204:dbl[][])  [unwired: 2 in]
        n88 = local write "Timings"(w204) -> ()
        n89 = Wait (ms)(milliseconds to wait="get variable interval (ms)") -> ()  [unwired: 1 out]
      }
    }
  }
  n90 = stacked-sequence {
    seq-local: [w209 _ _ _ _] -> [_ _ w332 _ _]
    tunnel: w7 -> [_ _ _ _ _]
    tunnel: [_ _ _ _ w910] -> w9
    tunnel: w1 -> [_ _ w336 _ _]
    tunnel: w5 -> [w210 _ _ _ _]
    tunnel: w3 -> [_ _ w335 w885 _]
    tunnel: w2 -> [_ _ w334 _ _]
    frame #0 {
      # "Initialize instruments and collect informations"
      # "Load experiment file"
      n91 = Tick Count (ms)() -> (millisecond timer value=w209:u32)
      n92 = Unbundle By Name(w210) -> ("Inst_parameters.Inst_array"=w218:T12, "Read out instrument bools"=w217:u64[][], "sweep_list"=w215:string[], "Sweep instrument bools"=w214:u64[][])
      n93 = Index Array(array=w214, index (col)=0) -> (element=w213:u64[])  [unwired: 1 in]
      n94 = Index Array(array=w217, index (col)=0) -> (element=w216:u64[])  [unwired: 1 in]
      n95 = call "Insts_init.vi"("Initialize sweep instruments ??"=w213, "sweep_list"=w215, "Initialize readout instruments??"=w216, "Inst_array"=w218) -> ("Sweep inst parameters"=→"Sweep inst info":T19, "Readout inst parameters"=→"Readout parameters":T19)
    }
    frame #1 {
      w223 = 0
      w222 = FALSE
      n96 = local write "start read vals"(TRUE) -> ()
      n97 = local read "Exp_params"() -> (w230:T15)
      n98 = Unbundle By Name(w230) -> ("Experimental bool list"=w235:bool[], "Inst_parameters.Inst_array"=w229:T12, "Sweep instrument bools"=w225:u64[][])
      n99 = Index Array(array=w225, index (col)=w223) -> (element=w224:u64[])  [unwired: 1 in]
      n100 = for {
        tunnel: w229 -> [w260] mode=indexing
        shift-right: [w262] -> w231
        shift-left: w222 -> [w263]
        shift-right: [w259] -> w236
        shift-left: "" -> [w261]
        shift-right: [w257] -> w228
        shift-left: w222 -> [w258]
        tunnel: w224 -> [w256]
        shift-right: [w253] -> _
        shift-left: w223 -> [w254]
        shift-right: [w251] -> w221
        shift-left: w222 -> [w252]
        # "Check DAC is used or not"
        n101 = Unbundle By Name(w260) -> ("Kind"=w255:u16)
        n102 = case shown="100, Default" w255 {
          tunnel: w263 -> [w268 w273 w278 w283 _ _ _ _ w325 w329]
          tunnel: [w268 w273 w278 w283 TRUE w298 TRUE TRUE w325 w329] -> w262
          tunnel: w261 -> [w267 w272 w277 w282 _ _ _ _ w324 w330]
          tunnel: w260 -> [_ _ _ _ w291 w302 w310 w319 _ _]
          tunnel: [w267 w272 w277 w282 w288 w299 w307 w316 w324 w330] -> w259
          tunnel: w258 -> [w266 w271 w276 w281 w287 _ w306 w315 w323 w331]
          tunnel: [w266 w271 w276 w281 w287 w298 w306 w315 w323 w331] -> w257
          tunnel: w256 -> [_ _ _ _ _ w296 _ _ _ _]
          tunnel: w254 -> [w265 w270 w275 w280 w286 w295 w304 w314 w322 w327]
          tunnel: [w265 w270 w275 w280 w285 w297 w305 w313 w322 w328] -> w253
          tunnel: [w264 w269 w274 w279 w284 w293 w303 w312 w321 w326] -> w251
          tunnel: w252 -> [w264 w269 w274 w279 w284 _ w303 w312 w321 w326]
          frame 0 {
          }
          frame 1 {
          }
          frame 2 {
          }
          frame 3 {
          }
          frame 4 {
            # "DAC"
            n103 = Unbundle By Name(w291) -> ("Strings"=w290:string[])
            n104 = Index Array(array=w290, index=1) -> (element=w288:string)
            n105 = Increment(x=w286) -> (x+1=w285:i32)
          }
          frame 5 {
            w298 = TRUE
            # "DAC lock-in"
            n106 = Unbundle By Name(w302) -> ("Strings"=w301:string[])
            n107 = Index Array(array=w296, index=w295) -> (element=w294:u64)
            n108 = Index Array(array=w301, index=1) -> (element=w299:string)
            n109 = Not Equal To 0?(x=w294) -> (x != 0?=w293:bool)
            n110 = Increment(x=w295) -> (x+1=w297:i32)
            "DAC_lock-in_info" <- w302
          }
          frame 9 {
            # "Fast sequence"
            n111 = Unbundle By Name(w310) -> ("Strings"=w309:string[])
            n112 = Index Array(array=w309, index=1) -> (element=w307:string)
            n113 = Increment(x=w304) -> (x+1=w305:i32)
          }
          frame 10 {
            # "Fast sequence slot"
            n114 = Unbundle By Name(w319) -> ("Strings"=w318:string[])
            n115 = Index Array(array=w318, index=1) -> (element=w316:string)
            n116 = Increment(x=w314) -> (x+1=w313:i32)
          }
          frame 12 {
            # "DSP lock-in readout"
          }
          frame 100, Default {
            n117 = Increment(x=w327) -> (x+1=w328:i32)
          }
        }
      }
      n118 = Replace Array Subset(array=w235, new element=w231, index=1) -> (w233:bool[])
      n119 = Bundle By Name(cluster=w230, "Experimental bool list"=w233) -> (w232:T15)
      n120 = case shown="True" w231 {
        tunnel: w236 -> [_ w250]
        tunnel: w232 -> [w244 w249]
        tunnel: [w244 w248] -> w227
        tunnel: w229 -> [_ w245]
        frame False {
        }
        frame True {
          # "Initialize used busses"
          # "Get FPGA reference if DAC is used."
          # "Open FPGA"
          n121 = call "OpenFPGARef.vi"("IP Address"=w250) -> ("FPGA VI Reference Out"=w247:T14)
          n122 = call "DAC_set_use_buses.vi"("FPGA Ref"=w247, "Use FPGA?"=TRUE, "Inst_array"=w245) -> ()  [unwired: 1 out]
          n123 = Bundle By Name(cluster=w249, "FPGA Ref"=w247) -> (w248:T15)
        }
      }
      n124 = case shown="True" w228 {
        tunnel: w227 -> [_ w241]
        tunnel: w221 -> [_ w238]
        frame False {
        }
        frame True {
          # "DAC lock in init"
          n125 = local read "DAC_lock-in_info"() -> (w239:T4)
          n126 = Unbundle By Name(w241) -> ("FPGA Ref"=w240:T14)
          n127 = case shown="True" w238 {
            tunnel: w240 -> [_ w243]
            tunnel: w239 -> [_ w242]
            frame False {
            }
            frame True {
              # "check sweep inst\nbool"
              n128 = call "DAC_lock_in_init.vi"("Inst info"=w242, "FPGA VI Reference In"=w243) -> ()  [unwired: 1 in]
            }
          }
        }
      }
      n129 = local write "Exp_params"(w227) -> ()
    }
    frame #2 {
      # "Check mode"
      n130 = local read "Exp_params"() -> (w339:T15)
      n131 = Unbundle By Name(w339) -> ("Inst_parameters.fast_mode"=w338:u8[])
      n132 = call "Sweep_mode.vi"("fast_mode"=w338) -> ("ramp?"=w337:bool, "Sweep mode"=w333:enum16{"Normal sweep", "Fast sweep"})  [unwired: 1 in]
      n133 = case shown="\"Normal sweep\", Default" w333 {
        tunnel: u64 0 -> [w360 w541]
        tunnel: w339 -> [w356 w531]
        tunnel: w337 -> [_ w533]
        tunnel: w334 -> [w347 w529]
        tunnel: w336 -> [w346 w528]
        tunnel: w335 -> [w343 w525]
        tunnel: w332 -> [w341 w523]
        frame "Normal sweep", Default {
          n134 = Unbundle By Name(w356) -> ("Initial move"=w345:T3, "sweep_dim"=w355:u64[], "ExpFilePath"=w342:path, "sweep_list"=w354:string[], "Inst_parameters.Wait_times"=w353:u64[], "readout_list"=w352:string[], "FPGA Ref"=w350:T14, "Experimental bool list"=w349:bool[], "Inst_parameters.Inst_array"=w344:T12)
          n135 = local read "Readout parameters"() -> (w358:T12)
          n136 = local read "Sweep inst info"() -> (w357:T12)
          n137 = Index Array(array=w349, index=1) -> (element=w348:bool)
          n138 = stacked-sequence {
            seq-local: [w361 _ _] -> [_ w382 _]
            seq-local: [_ w383 _] -> [_ _ w399]
            tunnel: w360 -> [_ _ w416]
            tunnel: 0 -> [_ _ w415]
            tunnel: w358 -> [_ _ w414]
            tunnel: w357 -> [_ _ w413]
            tunnel: w355 -> [w372 _ w412]
            tunnel: w354 -> [_ _ w411]
            tunnel: w353 -> [w370 _ w410]
            tunnel: w352 -> [_ _ w409]
            tunnel: w350 -> [w369 w390 w408]
            tunnel: w348 -> [w367 w389 w407]
            tunnel: w347 -> [_ _ w406]
            tunnel: w346 -> [_ _ w405]
            tunnel: w345 -> [w371 _ _]
            tunnel: w344 -> [w368 w391 _]
            tunnel: w343 -> [w366 _ w404]
            tunnel: w342 -> [_ w388 _]
            tunnel: w341 -> [w362 _ _]
            frame #0 {
              # "Perform initial movement"
              # "Collect information of the instruments\nto be moved at the beggining."
              # "Wait after initial movement"
              n139 = local read "Timings"() -> (w364:dbl[][])
              n140 = Tick Count (ms)() -> (millisecond timer value=w361:u32)
              n141 = call "Timer.vi"("index"=4, "Timings in"=w364, "t1"=w362, "t2"=w361) -> ("Timings out"=w365:dbl[][])  [unwired: 2 in]
              n142 = Index Array(array=w370, index=0) -> (element=w374:u64)
              n143 = local write "Timings"(w365) -> ()
              n144 = call "Select_inst_info.vi"("Inst_parameters.Inst_array"=w368, "Initial move"=w371) -> ("Inst_parameters.Inst_array 2"=w373:T12)
              n145 = flat-sequence {
                tunnel: w371 -> [w378]
                tunnel: w369 -> [w380]
                tunnel: w373 -> [w379]
                tunnel: w367 -> [w377]
                tunnel: w366 -> [w376]
                tunnel: w374 -> [w381]
                frame #0 {
                  # "Move"
                  n146 = call "Move.vi"("Points"=w378, "Sweep inst info"=w379, "FPGA Ref"=w380, "Use FPGA?"=w377, "WorkFilePath"=w376) -> ()  [unwired: 5 in, 1 out]
                }
                frame #1 {
                  # "Initial wait (ms)"
                  n147 = Wait (ms)(milliseconds to wait=w381) -> ()  [unwired: 1 out]
                }
              }
              "sweep_dim" <- w372
            }
            frame #1 {
              # "Register value of all the instruments before the measurement"
              n148 = local read "Timings"() -> (w385:dbl[][])
              n149 = Tick Count (ms)() -> (millisecond timer value=w383:u32)
              n150 = call "Timer.vi"("index"=7, "Timings in"=w385, "t1"=w382) -> ("Timings out"=w386:dbl[][])  [unwired: 3 in]
              n151 = local write "Timings"(w386) -> ()
              n152 = call "GetTempFilePath.vi"("ExpFilePath"=w388) -> ("Temp file path"=w387:path)
              n153 = case shown="False" w389 {
                tunnel: w390 -> [_ w398]
                tunnel: [w394 w397] -> w392
                frame False {
                  w396 = 8
                  n154 = Initialize Array(0.0, w396, w396) -> (w394:dbl[][])
                }
                frame True {
                  n155 = call "DAC_current_values.vi"("FPGA Ref"=w398) -> ("DAC values"=w397:sgl[][])
                }
              }
              n156 = call "Get_values.vi"("DAC values"=w392, "Inst_array"=w391, "Temp file path"=w387) -> ("Initial positions"=→"Initial positions":T3)
            }
            frame #2 {
              n157 = while {
                shift-right: [w442] -> _
                shift-left: w416 -> [w428]
                shift-right: [w436] -> _
                shift-left: w415 -> [w437]
                tunnel: w414 -> [w434]
                tunnel: w413 -> [w427]
                tunnel: w412 -> [w433]
                tunnel: w411 -> [w422]
                tunnel: w410 -> [w432]
                tunnel: w409 -> [w431]
                tunnel: w408 -> [w430]
                tunnel: w407 -> [w429]
                tunnel: w406 -> [w426]
                tunnel: w405 -> [w425]
                tunnel: w404 -> [w420]
                stop <- w441 stop-if-true
                # "Seep indexes"
                # "Stop if stop button is pushed or\nindex reaches the sweep dimension."
                n158 = Array Size(array=w422) -> (size(s)=w423:i32)
                n159 = Not Equal To 0?(x=w423) -> (x != 0?=w421:bool)
                n160 = case shown="True" w421 {
                  tunnel: w425 -> [_ w445]
                  tunnel: [cluster{string, "data":u64, dbl}[] [{"None", "data"=100, 0.0}] w444] -> w424
                  frame False {
                  }
                  frame True {
                    n161 = Dequeue Element(queue=w445) -> (element=w444:cluster{string, "data":u64, dbl}[])  [unwired: 2 in, 3 out]
                  }
                }
                n162 = call "Count2Indexes.vi"("sweep_dim"=w433, "Count"=w428) -> ("Indexes"=w439:u64[])
                "Indexes" <- w439
                n163 = Tick Count (ms)() -> (millisecond timer value=w418:u32)
                n164 = stacked-sequence {
                  seq-local: [_ _ _ w480 _ _ _] -> [_ _ _ _ w492 w497 _]
                  seq-local: [_ _ w455 _ _ _ _] -> [_ _ _ _ w486 _ _]
                  seq-local: [_ _ _ _ w485 _ _] -> [_ _ _ _ _ _ w518]
                  tunnel: w427 -> [w449 _ _ _ _ _ _]
                  tunnel: w432 -> [_ w454 w460 w483 _ _ _]
                  tunnel: w434 -> [_ _ _ w481 _ _ _]
                  tunnel: w439 -> [w448 _ w463 _ _ w493 w522]
                  tunnel: w433 -> [_ _ _ _ _ w498 w511]
                  tunnel: w431 -> [_ _ _ _ _ _ _]
                  tunnel: [_ _ _ _ _ _ w511] -> w419
                  tunnel: [_ _ _ _ _ _ w522] -> w417
                  tunnel: w437 -> [_ _ w462 _ _ _ _]
                  tunnel: [_ _ w461 _ _ _ _] -> w436
                  tunnel: w430 -> [w451 _ _ _ _ _ _]
                  tunnel: w429 -> [w450 _ _ _ _ _ _]
                  tunnel: w428 -> [_ _ _ _ _ _ w510]
                  tunnel: w426 -> [_ _ _ _ w487 _ _]
                  tunnel: w424 -> [w446 _ _ _ _ w495 _]
                  tunnel: w420 -> [w447 _ _ _ _ _ _]
                  tunnel: w418 -> [_ _ w456 _ _ _ w514]
                  frame #0 {
                    # "Move to the position"
                    n165 = call "Move.vi"("Points"=w446, "Sweep inst info"=w449, "FPGA Ref"=w451, "Use FPGA?"=w450, "WorkFilePath"=w447, "Indexes"=w448) -> ()  [unwired: 4 in, 1 out]
                  }
                  frame #1 {
                    # "Wait before measurement"
                    n166 = Index Array(array=w454, index=1) -> (element=w452:u64)
                    n167 = Wait (ms)(milliseconds to wait=w452) -> ()  [unwired: 1 out]
                  }
                  frame #2 {
                    # "Extra wait time\nwhen we step."
                    # "Wait after step movement"
                    n168 = Array Size(array=w463) -> (size(s)=w465:i32)
                    n169 = Tick Count (ms)() -> (millisecond timer value=w455:u32)
                    n170 = Greater?(x=w465, y=1) -> (0:w466:bool)
                    n171 = case shown="True" w466 {
                      tunnel: w463 -> [_ w474]
                      tunnel: w462 -> [w467 w471]
                      tunnel: [w467 w470] -> w461
                      tunnel: w460 -> [_ w468]
                      frame False {
                      }
                      frame True {
                        n172 = Index Array(array=w474, index=1) -> (element=w469:u64)
                        n173 = Equal?(x=w469, y=w471) -> (x = y?=w472:bool)
                        n174 = case shown="False" w472 {
                          tunnel: w471 -> [_ w479]
                          tunnel: [w478 w479] -> w470
                          tunnel: w469 -> [w478 _]
                          tunnel: w468 -> [w477 _]
                          frame False {
                            n175 = Index Array(array=w477, index=3) -> (element=w475:u64)
                            n176 = Wait (ms)(milliseconds to wait=w475) -> ()  [unwired: 1 out]
                          }
                          frame True {
                          }
                        }
                      }
                    }
                    n177 = local read "Timings"() -> (w458:dbl[][])
                    n178 = call "Timer.vi"("index"=10, "Timings in"=w458, "t1"=w456, "t2"=w455) -> ("Timings out"=w457:dbl[][])  [unwired: 2 in]
                    n179 = local write "Timings"(w457) -> ()
                  }
                  frame #3 {
                    # "Readout data"
                    n180 = Index Array(array=w483, index=2) -> (element=w482:u64)
                    n181 = call "Read.vi"("Readout parameters"=w481, "Integration time (ms)"=w482) -> ("Data"=w480:dbl[])  [unwired: 1 in]
                  }
                  frame #4 {
                    # "Save data to the file"
                    n182 = Build Array(w492) -> (w491:dbl[][])
                    n183 = local write "Temp data"(w491) -> ()
                    n184 = Enqueue Element(queue=w487, element=w491) -> ()  [unwired: 2 in, 3 out]
                    n185 = local read "Timings"() -> (w489:dbl[][])
                    n186 = Tick Count (ms)() -> (millisecond timer value=w485:u32)
                    n187 = call "Timer.vi"("index"=14, "Timings in"=w489, "t1"=w486, "t2"=w485) -> ("Timings out"=w488:dbl[][])  [unwired: 2 in]
                    n188 = local write "Timings"(w488) -> ()
                  }
                  frame #5 {
                    n189 = local read "Plot parameters"() -> (w494:T2)
                    n190 = Unbundle By Name(w494) -> ("Disable plot"=w496:bool)
                    n191 = case shown="False" w496 {
                      tunnel: w498 -> [w504 _]
                      tunnel: w497 -> [w502 _]
                      tunnel: w495 -> [w508 _]
                      tunnel: w493 -> [w505 _]
                      frame False {
                        # "Add data to plot queue"
                        n192 = Build Array(w502) -> (w499:dbl[][])
                        n193 = local read "Plot parameters"() -> (w506:T2)
                        n194 = Array Size(array=w502) -> (size(s)=w501:i32)
                        n195 = Array Size(array=w499) -> (size(s)=w500:i32[])
                        n196 = Index Array(array=w499, index (row)=w501) -> ()  [unwired: 1 in, 1 out]
                        n197 = Index Array(array=w500) -> ()  [unwired: 1 in, 1 out]
                        n198 = call "Plot_add_to_buffer.vi"("Plot parameters in"=w506, "fast mode"=enum16{"normal sweep", "fast sweep"}."normal sweep", "Points"=w508, "new_data"=w499, "sweep_dim"=w504, "Indexes"=w505) -> ("Plot parameters out"=w507:T2)  [unwired: 1 in]
                        n199 = local write "Plot parameters"(w507) -> ()
                      }
                      frame True {
                      }
                    }
                  }
                  frame #6 {
                    # "Sweep counter check"
                    n200 = local read "Timings"() -> (w516:dbl[][])
                    n201 = local read "Timings"() -> (w520:dbl[][])
                    n202 = Tick Count (ms)() -> (millisecond timer value=w517:u32)
                    n203 = Tick Count (ms)() -> (millisecond timer value=w519:u32)
                    n204 = call "Timer.vi"("index"=9, "Timings in"=w516, "t1"=w514, "t2"=w517) -> ("Timings out"=w512:dbl[][])  [unwired: 2 in]
                    n205 = call "Timer.vi"("index"=2, "Timings in"=w520, "t1"=w518, "t2"=w519) -> ("Timings out"=w513:dbl[][])  [unwired: 2 in]
                    n206 = local write "Timings"(w512) -> ()
                    n207 = local write "Timings"(w513) -> ()
                    n208 = call "RemainingTime.vi"("Timings"=w512, "sweep_dim"=w511, "Count"=w510) -> ("Remaning time (min)"=w509:dbl)
                    n209 = local write "Remaning time (min)"(w509) -> ()
                  }
                }
                n210 = Decrement(x=w419) -> (x-1=w435:u64[])
                n211 = Equal?(x=w417, y=w435) -> (x = y?=w438:bool)
                n212 = local read "Stop"() -> (w440:bool)
                n213 = Increment(x=w428) -> (x+1=w442:u64)
                n214 = Or(x=w438, y=w440) -> (x .or. y?=w441:bool)
              }
              n215 = local read "Timings"() -> (w401:dbl[][])
              n216 = Tick Count (ms)() -> (millisecond timer value=w403:u32)
              n217 = call "Timer.vi"("index"=6, "Timings in"=w401, "t1"=w399, "t2"=w403) -> ("Timings out"=w400:dbl[][])  [unwired: 2 in]
              n218 = local write "Timings"(w400) -> ()
            }
          }
        }
        frame "Fast sweep" {
          (unwired) 0
          # "Number of points to keep"
          # "File ref"
          # "Type of reding instrument\nex.) ADC, K2000, Lecroy\n(We asuume that we only\nuse 1 kind of an instrument\nat a time. If this condition is\nnot met, error comes out.)"
          # "Number of point to acquire"
          # "FPGA ref"
          n219 = Unbundle By Name(w531) -> ("Initial move"=w527:T3, "FPGA Ref"=w532:T14, "Inst_parameters.ConfigFilePath"=w534:path, "sweep_dim"=w535:u64[], "sweep_list"=w538:string[], "readout_list"=w537:string[], "Inst_parameters.Wait_times"=w536:u64[], "Experimental bool list"=w530:bool[], "Inst_parameters.Inst_array"=w526:T12, "ExpFilePath"=w524:path)
          n220 = local read "Sweep inst info"() -> (w539:T12)
          n221 = local read "Readout parameters"() -> (w540:T12)
          n222 = stacked-sequence {
            seq-local: [_ w572 _ _ _ _ _] -> [_ _ w643 _ _ w722 _]
            seq-local: [w544 _ _ _ _ _ _] -> [_ w571 w641 _ _ w726 w876]
            seq-local: [_ w565 _ _ _ _ _] -> [_ _ _ _ _ w721 _]
            seq-local: [_ w560 _ _ _ _ _] -> [_ _ w635 _ _ _ _]
            seq-local: [_ _ w636 _ _ _ _] -> [_ _ _ w674 _ _ _]
            seq-local: [_ _ _ w675 _ _ _] -> [_ _ _ _ w697 _ _]
            seq-local: [_ _ _ _ w698 _ _] -> [_ _ _ _ _ w716 _]
            tunnel: w541 -> [_ _ _ _ _ w734 _]
            tunnel: w540 -> [_ _ w640 _ _ _ _]
            tunnel: w539 -> [_ _ _ _ _ w731 _]
            tunnel: w538 -> [_ _ _ _ _ w732 _]
            tunnel: w537 -> [_ _ _ _ _ w728 _]
            tunnel: w536 -> [_ _ _ w687 _ w730 _]
            tunnel: w535 -> [_ _ _ w680 _ w733 _]
            tunnel: w534 -> [w550 _ _ _ _ _ _]
            tunnel: w533 -> [_ w570 w642 _ _ w729 _]
            tunnel: w532 -> [w545 _ _ w683 w707 _ _]
            tunnel: w531 -> [w549 _ _ _ _ _ _]
            tunnel: w530 -> [w547 _ _ w685 w706 w727 _]
            tunnel: w529 -> [_ _ _ _ _ w725 _]
            tunnel: w528 -> [_ _ _ _ _ w724 _]
            tunnel: w527 -> [_ _ _ w682 _ _ _]
            tunnel: w526 -> [_ _ _ w681 w705 _ _]
            tunnel: w525 -> [_ _ _ w679 _ w723 _]
            tunnel: w524 -> [_ _ _ _ w704 _ _]
            tunnel: w523 -> [_ w561 _ _ _ _ _]
            frame #0 {
              # "Get fast sequence inforamtion"
              n223 = call "Get_fast_seq_info.vi"("ConfigFilePath"=w550) -> ("Fast sequence parameters"=w543:T11)
              "Fast sequence parameters" <- w543
              n224 = Unbundle By Name(w543) -> ("IP address"=w542:string)
              n225 = Index Array(array=w547, index=1) -> (element=w546:bool)
              n226 = case shown="False" w546 {
                tunnel: w549 -> [w558 _]
                tunnel: w547 -> [w557 _]
                tunnel: w545 -> [_ w559]
                tunnel: [w552 w559] -> w544
                tunnel: w542 -> [w551 _]
                frame False {
                  # "Update use FPGA status here if it is FALSE before"
                  n227 = call "OpenFPGARef.vi"("IP Address"=w551) -> ("FPGA VI Reference Out"=w552:T14)
                  n228 = Replace Array Subset(array=w557, new element=TRUE, index=1) -> (w554:bool[])
                  n229 = Bundle By Name(cluster=w558, "Experimental bool list"=w554, "FPGA Ref"=w552) -> (w553:T15)
                  n230 = local write "Exp_params"(w553) -> ()
                }
                frame True {
                }
              }
            }
            frame #1 {
              # "Initialize the fast sequence"
              n231 = local read "Timings"() -> (w562:dbl[][])
              n232 = local read "Fast sequence parameters"() -> (w569:T11)
              n233 = call "Fast_seq_init.vi"("FPGA Ref"=w571, "Ramp?"=w570, "Fast sequence parameters 2"=w569) -> ()
              n234 = Tick Count (ms)() -> (millisecond timer value=w560:u32)
              n235 = Unbundle By Name(w569) -> ("Sequence size"=w574:u64, "Sample count"=w573:u64, "Start ramp at"=w566:u64, "fastseq"=w568:T20, "Fast-seq-divider"=w567:u64)
              n236 = call "Timer.vi"("index"=4, "Timings in"=w562, "t1"=w561, "t2"=w560) -> ("Timings out"=w563:dbl[][])  [unwired: 2 in]
              n237 = local write "Timings"(w563) -> ()
              n238 = case shown="True" w570 {
                tunnel: [w575 w577] -> w572
                tunnel: w574 -> [_ w580]
                tunnel: w573 -> [w575 _]
                tunnel: w568 -> [_ w587]
                tunnel: w567 -> [_ w585]
                tunnel: w566 -> [_ w581]
                tunnel: [w575 w576] -> w565
                frame False {
                }
                frame True {
                  # "minimum size : trigger + ramp + jump"
                  # "convert pre-ramp sequence to additional points"
                  # "jump next steps"
                  n239 = Subtract(x=w580, y=w581) -> (x-y=w579:u64)
                  n240 = Subtract(x=w579, y=2) -> (x-y=w576:u64)
                  n241 = for {
                    N: w580 -> [_]
                    tunnel: w587 -> [w596] mode=indexing
                    shift-right: [w588] -> w583
                    shift-left: 0.0 -> [w599]
                    tunnel: w585 -> [w597]
                    shift-right: [w593] -> _
                    shift-left: 0 -> [w590]
                    i -> [w592]
                    n242 = Unbundle By Name(w596) -> ("use"=w598:T5, "timing"=w595:T9, "slot#"=w594:T10)
                    n243 = Greater?(x=w590, y=0) -> (0:w589:bool)
                    n244 = case shown="False" w589 {
                      tunnel: w599 -> [w608 w632]
                      tunnel: [w607 w632] -> w588
                      tunnel: w598 -> [w606 _]
                      tunnel: w597 -> [w605 _]
                      tunnel: w595 -> [w604 _]
                      tunnel: w594 -> [w603 _]
                      tunnel: w590 -> [w602 w634]
                      tunnel: [w601 w633] -> w593
                      tunnel: w592 -> [w600 _]
                      frame False {
                        n245 = case shown="\"timing\"" w606 {
                          tunnel: w608 -> [w611 w619 w625 w626]
                          tunnel: [w610 w616 w625 w626] -> w607
                          tunnel: w605 -> [_ w620 _ _]
                          tunnel: w604 -> [_ w614 _ _]
                          tunnel: w603 -> [_ _ _ w629]
                          tunnel: w602 -> [w609 w615 w624 w631]
                          tunnel: [w609 w615 w624 w630] -> w601
                          tunnel: w600 -> [_ _ _ w628]
                          frame "DAC", Default {
                            n246 = Increment(x=w611) -> (x+1=w610:dbl)
                          }
                          frame "timing" {
                            # "actual timing is 5% larger"
                            # "equivalent number\nof points"
                            # "time per point"
                            n247 = Multiply(x=w614, y=1.05) -> (x*y=w613:dbl)
                            n248 = Multiply(x=w620, y=0.4501) -> (x*y=w622:dbl)
                            n249 = Divide(x=w622, y=1000.0) -> (x/y=w618:dbl)
                            n250 = Divide(x=w613, y=w618) -> (x/y=w617:dbl)
                            n251 = Add(x=w617, y=w619) -> (x+y=w616:dbl)
                          }
                          frame "triggers" {
                            # "triggers are not\ntaken into account"
                          }
                          frame "jump" {
                            # "N next steps will be jumped"
                            n252 = Subtract(x=w629, y=w628) -> (x-y=w627:i32)
                            n253 = Add(x=w631, y=w627) -> (x+y=w630:i32)
                          }
                        }
                      }
                      frame True {
                        # "step is jumped"
                        n254 = Decrement(x=w634) -> (x-1=w633:i32)
                      }
                    }
                  }
                  n255 = Round To Nearest(number=w583) -> (nearest integer value=w582:dbl)
                  n256 = To Unsigned Quad Integer(1:w582) -> (0:w577:u64)
                }
              }
            }
            frame #2 {
              # "Configure and initialize voltmeters for fast ramp"
              n257 = local read "Timings"() -> (w638:dbl[][])
              n258 = Tick Count (ms)() -> (millisecond timer value=w636:u32)
              n259 = call "Timer.vi"("index"=5, "Timings in"=w638, "t1"=w635, "t2"=w636) -> ("Timings out"=w639:dbl[][])  [unwired: 2 in]
              n260 = local write "Timings"(w639) -> ()
              n261 = for {
                tunnel: w640 -> [w649] mode=indexing
                tunnel: w643 -> [w648]
                tunnel: w642 -> [w647]
                tunnel: w641 -> [w646]
                tunnel: w640 -> [w645]
                i -> [w644]
                n262 = Unbundle By Name(w649) -> ("Kind"=w650:u16)
                n263 = case shown="0" w650 {
                  tunnel: w649 -> [w653 w662 _ w672 _]
                  tunnel: w648 -> [w658 w661 _ w670 _]
                  tunnel: w647 -> [w659 _ _ w671 _]
                  tunnel: w646 -> [_ w660 _ w673 _]
                  tunnel: w645 -> [w655 _ _ _ _]
                  tunnel: w644 -> [w654 _ _ _ _]
                  frame 0 {
                    # "Update take out\nand sample per\nchannel"
                    # "ADC"
                    n264 = local read "Fast sequence parameters"() -> (w657:T11)
                    n265 = Unbundle By Name(w657) -> ("Fast-seq-divider"=w656:u64)
                    n266 = call "ADC_config_fastsweep.vi"("Inst_parameter"=w653, "Fast sequence size"=w658, "fast sequence divider"=w656, "Ramp?"=w659) -> ("Inst_parameter out"=w651:T4)  [unwired: 1 in]
                    n267 = Replace Array Subset(array=w655, new element=w651, index=w654) -> (w652:T12)
                    n268 = local write "Readout parameters"(w652) -> ()
                  }
                  frame 1 {
                    # "K2000"
                    n269 = stacked-sequence {
                      tunnel: w662 -> [w665 w669]
                      tunnel: w661 -> [w664 _]
                      tunnel: w660 -> [w663 _]
                      frame #0 {
                        n270 = call "K2000_config_fastsweep.vi"("Readout_inst_parameters"=w665, "readings"=w664) -> ()  [unwired: 1 in, 1 out]
                        n271 = call "DAC_set_stop-sample-count.vi"("FPGA VI Reference In"=w663) -> ()  [unwired: 1 in, 10 out]
                      }
                      frame #1 {
                        n272 = Unbundle By Name(w669) -> ("Strings"=w668:string[])
                        n273 = Index Array(array=w668, index=1) -> (element=w666:string)
                        n274 = call "K2000_init_fastseq.vi"("GPIB address"=w666) -> ()
                      }
                    }
                  }
                  frame 3 {
                    # "LeCroy"
                  }
                  frame 12 {
                    # "Lock-in"
                    n275 = call "DSP_init_fast_sweep.vi"("Sample count"=w670, "ramp?"=w671, "Inst info"=w672) -> ()  [unwired: 1 in]
                    n276 = call "DAC_set_stop-sample-count.vi"("FPGA VI Reference In"=w673) -> ()  [unwired: 1 in, 10 out]
                  }
                  frame 100, Default {
                  }
                }
              }
            }
            frame #3 {
              # "Perform initial movement"
              # "Collect information of the instruments\nto be moved at the beggining."
              # "Wait after initial movement"
              n277 = local write "sweep_dim"(w680) -> ()
              n278 = Index Array(array=w685, index=1) -> (element=w684:bool)
              n279 = local read "Timings"() -> (w677:dbl[][])
              n280 = Tick Count (ms)() -> (millisecond timer value=w675:u32)
              n281 = call "Timer.vi"("index"=6, "Timings in"=w677, "t1"=w674, "t2"=w675) -> ("Timings out"=w678:dbl[][])  [unwired: 2 in]
              n282 = local write "Timings"(w678) -> ()
              n283 = Index Array(array=w687, index=0) -> (element=w689:u64)
              n284 = call "Select_inst_info.vi"("Inst_parameters.Inst_array"=w681, "Initial move"=w682) -> ("Inst_parameters.Inst_array 2"=w688:T12)
              n285 = flat-sequence {
                tunnel: w682 -> [w693]
                tunnel: w683 -> [w695]
                tunnel: w688 -> [w694]
                tunnel: w684 -> [w692]
                tunnel: w679 -> [w691]
                tunnel: w689 -> [w696]
                frame #0 {
                  # "Move"
                  n286 = call "Move.vi"("Points"=w693, "Sweep inst info"=w694, "FPGA Ref"=w695, "Use FPGA?"=w692, "WorkFilePath"=w691) -> ()  [unwired: 5 in, 1 out]
                }
                frame #1 {
                  # "Initial wait (ms)"
                  n287 = Wait (ms)(milliseconds to wait=w696) -> ()  [unwired: 1 out]
                }
              }
            }
            frame #4 {
              # "Register value of all the instruments before the measurement"
              n288 = call "GetTempFilePath.vi"("ExpFilePath"=w704) -> ("Temp file path"=w703:path)
              n289 = local read "Timings"() -> (w700:dbl[][])
              n290 = Tick Count (ms)() -> (millisecond timer value=w698:u32)
              n291 = call "Timer.vi"("index"=7, "Timings in"=w700, "t1"=w697, "t2"=w698) -> ("Timings out"=w701:dbl[][])  [unwired: 2 in]
              n292 = local write "Timings"(w701) -> ()
              n293 = Index Array(array=w706, index=1) -> (element=w709:bool)
              n294 = case shown="True" w709 {
                tunnel: w707 -> [_ w715]
                tunnel: [w711 w714] -> w708
                frame False {
                  w713 = 8
                  n295 = Initialize Array(0.0, w713, w713) -> (w711:dbl[][])
                }
                frame True {
                  n296 = call "DAC_current_values.vi"("FPGA Ref"=w715) -> ("DAC values"=w714:sgl[][])
                }
              }
              n297 = call "Get_values.vi"("DAC values"=w708, "Inst_array"=w705, "Temp file path"=w703) -> ("Initial positions"=w702:T3)
              n298 = local write "Initial positions"(w702) -> ()
            }
            frame #5 {
              # "Measurement loop"
              n299 = while {
                shift-right: [w762] -> _
                shift-left: w734 -> [w749]
                tunnel: w733 -> [w759]
                tunnel: w732 -> [w742]
                tunnel: w731 -> [w748]
                tunnel: w730 -> [w757]
                tunnel: w729 -> [w756]
                tunnel: w722 -> [w755]
                tunnel: w728 -> [w754]
                tunnel: w727 -> [w752]
                tunnel: w726 -> [w751]
                tunnel: w725 -> [w747]
                tunnel: w724 -> [w746]
                tunnel: w723 -> [w741]
                tunnel: w721 -> [w739]
                tunnel: w722 -> [w738]
                stop <- w740 stop-if-true
                n300 = local read "Readout parameters"() -> (w750:T12)
                n301 = Array Size(array=w742) -> (size(s)=w744:i32)
                n302 = Not Equal To 0?(x=w744) -> (x != 0?=w743:bool)
                n303 = call "Count2Indexes.vi"("sweep_dim"=w759, "Count"=w749) -> ("Indexes"=w753:u64[])
                n304 = case shown="True" w743 {
                  tunnel: w746 -> [_ w765]
                  tunnel: [cluster{string, "data":u64, dbl}[] [{"None", "data"=100, 0.0}] w764] -> w745
                  frame False {
                  }
                  frame True {
                    n305 = Dequeue Element(queue=w765) -> (element=w764:cluster{string, "data":u64, dbl}[])  [unwired: 2 in, 3 out]
                  }
                }
                n306 = Tick Count (ms)() -> (millisecond timer value=w737:u32)
                n307 = stacked-sequence {
                  seq-local: [_ _ w784 _ _ _ _ _ _] -> [_ _ _ w801 _ w821 _ _ _]
                  seq-local: [_ _ _ _ w810 _ _ _ _] -> [_ _ _ _ _ _ w830 w850 _]
                  seq-local: [_ _ w778 _ _ _ _ _ _] -> [_ _ _ w797 _ _ _ _ _]
                  seq-local: [_ _ _ w796 _ _ _ _ _] -> [_ _ _ _ w804 _ _ _ _]
                  seq-local: [_ _ _ _ w803 _ _ _ _] -> [_ _ _ _ _ w817 _ _ _]
                  seq-local: [_ _ _ _ _ w816 _ _ _] -> [_ _ _ _ _ _ w825 _ _]
                  seq-local: [_ _ _ _ _ _ w823 _ _] -> [_ _ _ _ _ _ _ w844 _]
                  seq-local: [_ _ _ _ _ _ _ w843 _] -> [_ _ _ _ _ _ _ _ w867]
                  tunnel: w753 -> [w768 _ _ _ _ _ _ w852 w863]
                  tunnel: w759 -> [_ _ _ _ _ _ _ w851 w862]
                  tunnel: [_ _ _ _ _ _ _ _ w862] -> w736
                  tunnel: [_ _ _ _ _ _ _ _ w863] -> w758
                  tunnel: w748 -> [w769 _ _ _ _ _ _ _ _]
                  tunnel: w757 -> [_ w776 _ _ _ _ _ _ _]
                  tunnel: w756 -> [_ _ w786 _ _ _ w828 _ _]
                  tunnel: w755 -> [_ _ w785 _ w815 _ _ _ _]
                  tunnel: w750 -> [_ _ _ _ _ _ w831 _ _]
                  tunnel: w754 -> [_ _ _ _ _ _ _ _ _]
                  tunnel: w752 -> [w774 _ _ _ _ _ _ _ _]
                  tunnel: w751 -> [w771 _ w783 _ _ _ _ _ _]
                  tunnel: [w770 _ _ _ _ _ _ _ _] -> _
                  tunnel: w749 -> [_ _ _ _ _ _ _ _ w861]
                  tunnel: w747 -> [_ _ _ _ _ _ w829 _ _]
                  tunnel: w745 -> [w767 _ _ _ _ _ _ w849 _]
                  tunnel: w741 -> [w766 _ _ _ _ _ _ _ _]
                  tunnel: w739 -> [_ _ _ _ w809 _ _ _ _]
                  tunnel: w738 -> [_ _ _ _ w811 _ _ _ _]
                  tunnel: w737 -> [_ _ w779 _ _ _ _ _ w872]
                  frame #0 {
                    # "Move to the point"
                    n308 = Index Array(array=w774, index=1) -> (element=w773:bool)
                    n309 = call "Move.vi"("Points"=w767, "Sweep inst info"=w769, "FPGA Ref"=w771, "Use FPGA?"=w773, "WorkFilePath"=w766, "Indexes"=w768) -> ("FPGA VI Reference Out"=w770:T14)  [unwired: 4 in]
                  }
                  frame #1 {
                    # "Wait after step movement\n(For the fast sequence there is no wait\nbetween sweep measurement)"
                    n310 = Index Array(array=w776, index=3) -> (element=w775:u64)
                    n311 = Wait (ms)(milliseconds to wait=w775) -> ()  [unwired: 1 out]
                  }
                  frame #2 {
                    # "Start fast sequence at the new sweep"
                    n312 = local read "Timings"() -> (w781:dbl[][])
                    n313 = Tick Count (ms)() -> (millisecond timer value=w778:u32)
                    n314 = case shown="True" w786 {
                      tunnel: w785 -> [w789 w791]
                      tunnel: [w788 w793] -> w784
                      tunnel: w783 -> [w787 w794]
                      frame False {
                        n315 = call "DAC_set_stop-sample-count.vi"("sample count"=w789, "FPGA VI Reference In"=w787) -> ("FPGA VI Reference Out"=w788:T14)  [unwired: 9 out]
                      }
                      frame True {
                        n316 = Add(x=w791, y=0) -> (x+y=w792:u64)
                        n317 = call "fastseq_set_orders.vi"("FPGA VI Reference In"=w794, "sample count"=w792, "Enum"=T18."set ramp") -> ("FPGA VI Reference Out"=w793:T14)  [unwired: 2 in]
                      }
                    }
                    n318 = call "Timer.vi"("index"=10, "Timings in"=w781, "t1"=w779, "t2"=w778) -> ("Timings out"=w780:dbl[][])  [unwired: 2 in]
                    n319 = local write "Timings"(w780) -> ()
                  }
                  frame #3 {
                    # "Start fast sequence"
                    n320 = local read "Timings"() -> (w799:dbl[][])
                    n321 = Tick Count (ms)() -> (millisecond timer value=w796:u32)
                    n322 = call "Timer.vi"("index"=11, "Timings in"=w799, "t1"=w797, "t2"=w796) -> ("Timings out"=w798:dbl[][])  [unwired: 2 in]
                    n323 = call "fastseq_set_orders.vi"("FPGA VI Reference In"=w801, "Enum"=T18."start") -> ()  [unwired: 3 in, 1 out]
                    n324 = local write "Timings"(w798) -> ()
                  }
                  frame #4 {
                    # "Read data"
                    n325 = local read "Readout parameters"() -> (w814:T12)
                    n326 = Subtract(x=w811, y=w809) -> (x-y=w808:u64)
                    n327 = call "Read_fastseq.vi"("Sequence size"=w815, "Readout parameters"=w814) -> ("measures"=w812:sgl[][], "Readout parameters out"=w813:T12)  [unwired: 2 in]
                    n328 = local read "Timings"() -> (w806:dbl[][])
                    n329 = Array Subset(array=w812, index (col)=w808, length (col)=w809) -> (w810:sgl[][])  [unwired: 2 in]
                    "Temp data" <- w810
                    n330 = Tick Count (ms)() -> (millisecond timer value=w803:u32)
                    n331 = local write "Readout parameters"(w813) -> ()
                    n332 = call "Timer.vi"("index"=12, "Timings in"=w806, "t1"=w804, "t2"=w803) -> ("Timings out"=w805:dbl[][])  [unwired: 2 in]
                    n333 = local write "Timings"(w805) -> ()
                  }
                  frame #5 {
                    # "Stop fast sequence"
                    n334 = local read "Timings"() -> (w819:dbl[][])
                    n335 = call "fastseq_set_orders.vi"("FPGA VI Reference In"=w821, "Enum"=T18."stop") -> ()  [unwired: 3 in, 1 out]
                    n336 = Tick Count (ms)() -> (millisecond timer value=w816:u32)
                    n337 = call "Timer.vi"("index"=14, "Timings in"=w819, "t1"=w817, "t2"=w816) -> ("Timings out"=w818:dbl[][])  [unwired: 2 in]
                    n338 = local write "Timings"(w818) -> ()
                  }
                  frame #6 {
                    # "Save array data"
                    # "Clear buffer before going to next"
                    n339 = for {
                      tunnel: w831 -> [w835] mode=indexing
                      tunnel: w831 -> [w834]
                      tunnel: w828 -> [w832]
                      i -> [w833]
                      n340 = Unbundle By Name(w835) -> ("Kind"=w836:u16)
                      n341 = case shown="0" w836 {
                        tunnel: w835 -> [w840 w841 _]
                        tunnel: w834 -> [w839 _ _]
                        tunnel: w833 -> [w838 _ _]
                        tunnel: w832 -> [_ w842 _]
                        frame 0 {
                          n342 = call "ADC_clean_buffer_batch.vi"("Index"=w838, "Readout parameters in"=w839, "Inst_param_in"=w840) -> ("Readout parameters out"=w837:T12)
                          n343 = local write "Readout parameters"(w837) -> ()
                        }
                        frame 12 {
                          n344 = call "DSPClearBuffer.vi"("Inst info"=w841, "ramp?"=w842) -> ()  [unwired: 1 in]
                        }
                        frame 100, Default {
                        }
                      }
                    }
                    n345 = local read "Timings"() -> (w827:dbl[][])
                    n346 = Enqueue Element(queue=w829, element=w830) -> ()  [unwired: 2 in, 3 out]
                    n347 = Tick Count (ms)() -> (millisecond timer value=w823:u32)
                    n348 = call "Timer.vi"("index"=13, "Timings in"=w827, "t1"=w825, "t2"=w823) -> ("Timings out"=w826:dbl[][])  [unwired: 2 in]
                    n349 = local write "Timings"(w826) -> ()
                  }
                  frame #7 {
                    # "Add data to plot queue"
                    n350 = local read "Plot parameters"() -> (w853:T2)
                    n351 = local read "Timings"() -> (w846:dbl[][])
                    n352 = Tick Count (ms)() -> (millisecond timer value=w843:u32)
                    n353 = call "Timer.vi"("index"=15, "Timings in"=w846, "t1"=w844, "t2"=w843) -> ("Timings out"=w845:dbl[][])  [unwired: 2 in]
                    n354 = Unbundle By Name(w853) -> ("Disable plot"=w848:bool)
                    n355 = case shown="False" w848 {
                      tunnel: w852 -> [w858 _]
                      tunnel: w851 -> [w857 _]
                      tunnel: w850 -> [w854 _]
                      tunnel: w849 -> [w856 _]
                      frame False {
                        n356 = local read "Plot parameters"() -> (w860:T2)
                        n357 = call "Plot_add_to_buffer.vi"("Plot parameters in"=w860, "fast mode"=enum16{"normal sweep", "fast sweep"}."fast sweep", "Points"=w856, "new_data"=w854, "sweep_dim"=w857, "Indexes"=w858) -> ("Plot parameters out"=w859:T2)  [unwired: 1 in]
                        n358 = local write "Plot parameters"(w859) -> ()
                      }
                      frame True {
                      }
                    }
                    n359 = local write "Timings"(w845) -> ()
                  }
                  frame #8 {
                    # "meas loop time"
                    n360 = local read "Timings"() -> (w873:dbl[][])
                    n361 = local read "Timings"() -> (w869:dbl[][])
                    n362 = Tick Count (ms)() -> (millisecond timer value=w874:u32)
                    n363 = Tick Count (ms)() -> (millisecond timer value=w868:u32)
                    n364 = call "Timer.vi"("index"=9, "Timings in"=w873, "t1"=w872, "t2"=w874) -> ("Timings out"=w864:dbl[][])  [unwired: 2 in]
                    n365 = call "Timer.vi"("index"=2, "Timings in"=w869, "t1"=w867, "t2"=w868) -> ("Timings out"=w865:dbl[][])  [unwired: 2 in]
                    n366 = local write "Timings"(w864) -> ()
                    n367 = local write "Timings"(w865) -> ()
                    n368 = call "RemainingTime.vi"("Timings"=w864, "sweep_dim"=w862, "Count"=w861) -> ("Remaning time (min)"=→"Remaning time (min)":dbl)
                  }
                }
                n369 = local write "Indexes"(w753) -> ()
                n370 = Increment(x=w749) -> (x+1=w762:u64)
                n371 = local read "Stop"() -> (w735:bool)
                n372 = Decrement(x=w736) -> (x-1=w760:u64[])
                n373 = Equal?(x=w758, y=w760) -> (x = y?=w761:bool)
                n374 = Or(x=w761, y=w735) -> (x .or. y?=w740:bool)
              }
              n375 = local read "Timings"() -> (w720:dbl[][])
              n376 = Tick Count (ms)() -> (millisecond timer value=w717:u32)
              n377 = call "Timer.vi"("index"=8, "Timings in"=w720, "t1"=w716, "t2"=w717) -> ("Timings out"=w719:dbl[][])  [unwired: 2 in]
              n378 = local write "Timings"(w719) -> ()
            }
            frame #6 {
              # "Post sweep treatment for the readout instruments"
              # "Final wait and close ADC etc."
              n379 = local read "Readout parameters"() -> (w875:T12)
              n380 = call "DAC_wait_end-of-move.vi"("FPGA VI Reference In"=w876) -> ()  [unwired: 1 in, 10 out]
              n381 = for {
                tunnel: w875 -> [w877] mode=indexing
                n382 = Unbundle By Name(w877) -> ("Kind"=w878:u16)
                n383 = case shown="0" w878 {
                  tunnel: w877 -> [w884 _]
                  frame 0 {
                    w883 = 0
                    n384 = Unbundle By Name(w884) -> ("DAQmx take out list"=w881:refnum<k21>[])
                    n385 = Increment(x=w883) -> (x+1=w882:i32)
                    n386 = Index Array(array=w881, index=w883) -> (element=w880:refnum<k21>)
                    n387 = Index Array(array=w881, index=w882) -> (element=w879:refnum<k21>)
                    n388 = call <vilib>:"DAQmx Clear Task.vi"("task in"=w880) -> ()  [unwired: 14 in, 1 out]
                    n389 = call <vilib>:"DAQmx Clear Task.vi"("task in"=w879) -> ()  [unwired: 14 in, 1 out]
                  }
                  frame 100, Default {
                  }
                }
              }
            }
          }
        }
      }
    }
    frame #3 {
      # "Post measurement treatment (temporal because it is not so nice.)"
      # "Go back to the initial position if it is required."
      n390 = local read "Exp_params"() -> (w893:T15)
      n391 = Unbundle By Name(w893) -> ("Experimental bool list"=w894:bool[], "FPGA Ref"=w895:T14)
      n392 = Index Array(array=w894, index=0) -> (element=w896:bool)
      n393 = Unbundle By Name(w893) -> ("Inst_parameters.Inst_array"=w888:T12, "Read out instrument bools"=w889:u64[][], "Sweep instrument bools"=w892:u64[][])
      n394 = case shown="True" w896 {
        tunnel: w893 -> [_ w905]
        tunnel: w895 -> [_ w904]
        tunnel: w894 -> [_ w902]
        tunnel: w885 -> [_ w898]
        frame False {
        }
        frame True {
          # "Move"
          # "Get initial values of sweep"
          # "Go to initial position"
          n395 = Unbundle By Name(w905) -> ("sweep_dim"=w908:u64[], "sweep_list"=w907:string[])
          n396 = call "Count2Indexes.vi"("sweep_dim"=w908, "Count"=0) -> ("Indexes"=w899:u64[])
          n397 = local read "Sweep inst info"() -> (w900:T12)
          n398 = call "GetValueFromIndexes.vi"("sweep_list"=w907, "WorkFilePath"=w898, "Sweep inst info"=w900, "Indexes"=w899) -> ("Points"=w906:cluster{"name":string, "data":u64, "data":dbl}[])
          n399 = Index Array(array=w902, index=1) -> (element=w901:bool)
          n400 = call "Move.vi"("Points"=w906, "Sweep inst info"=w900, "FPGA Ref"=w904, "Use FPGA?"=w901, "WorkFilePath"=w898, "Indexes"=w899) -> ()  [unwired: 4 in, 1 out]
        }
      }
      n401 = Index Array(array=w892, index (col)=1) -> (element=w886:u64[])  [unwired: 1 in]
      n402 = Index Array(array=w889, index (col)=1) -> (element=w887:u64[])  [unwired: 1 in]
      n403 = call "Insts_post.vi"("Initialize sweep instruments ??"=w886, "Initialize readout instruments??"=w887, "Inst_array"=w888) -> ()  [unwired: 3 in]
    }
    frame #4 {
      n404 = local read "Indexes"() -> (w910:i32[])
      n405 = local read "Exp_params"() -> (w915:T15)
      n406 = Unbundle By Name(w915) -> ("Experimental bool list"=w913:bool[], "FPGA Ref"=w914:T14)
      n407 = Index Array(array=w913, index=1) -> (element=w912:bool)
      n408 = case shown="True" w912 {
        tunnel: w914 -> [_ w916]
        frame False {
        }
        frame True {
          # "Close FPGA"
          n409 = xnode "Close FPGA VI Reference"("FPGA VI Reference In"=w916) -> ()  [unwired: 1 in, 1 out]
        }
      }
    }
  }
  n410 = stacked-sequence {
    tunnel: w9 -> [w920 _ _]
    tunnel: w8 -> [w927 w948 _]
    tunnel: w2 -> [w929 _ _]
    tunnel: w1 -> [w928 _ _]
    frame #0 {
      # "Write final indexes of the sweep."
      n411 = call "GetTempFilePath.vi"("ExpFilePath"=w927) -> ("Temp file path"=w926:path)
      n412 = call <vilib>:"H5Fopen.vi"("mode (read-only)"=H5Fmode."open or create" ("mode"), "path"=w926) -> ("error out"=w919:errorcluster, "ref out"=w921:T13)  [unwired: 8 in]
      n413 = xnode "H5Awrite.xnode"("replace? (T)"=TRUE, "object name"="Param_list", "error in (no error)"=w919, "data"=w920, "attrib name"="sweep_index", "ref in"=w921) -> ("error out"=w918:errorcluster, "ref out"=w917:T13)  [unwired: 1 in, 1 out]
      n414 = call <vilib>:"H5Fclose.vi"("error in (no error)"=w918, "ref"=w917) -> ()  [unwired: 9 in, 1 out]
      n415 = Release Queue(queue=w928) -> ()  [unwired: 2 in, 3 out]
      n416 = Release Queue(queue=w929) -> ()  [unwired: 2 in, 3 out]
    }
    frame #1 {
      # "Finally copy temp file\nto actual file"
      n417 = Delete(path (use dialog)=w948) -> (error out=w950:errorcluster)  [unwired: 4 in, 2 out]
      n418 = call "GetTempFilePath.vi"("ExpFilePath"=w948) -> ("Temp file path"=w949:path)
      n419 = Unbundle By Name(w950) -> ("status"=w951:bool)
      n420 = case shown="True" w951 {
        tunnel: w949 -> [w952 _]
        tunnel: w948 -> [w954 _]
        frame False {
          n421 = call "repack-h5.vi"("dest"=w954, "source"=w952) -> ("error out"=w953:errorcluster)  [unwired: 1 in]
          n422 = Delete(path (use dialog)=w952, error in=w953) -> ()  [unwired: 3 in, 3 out]
        }
        frame True {
        }
      }
    }
    frame #2 {
      n423 = local write "Finish"(TRUE) -> ()
    }
  }
  n424 = while {
    stop <- w956 stop-if-true
    n425 = stacked-sequence {
      seq-local: [w957 _ _] -> [_ _ w1000]
      frame #0 {
        n426 = Tick Count (ms)() -> (millisecond timer value=w957:u32)
      }
      frame #1 {
        n427 = local read "Plot parameters"() -> (w958:T2)
        n428 = Unbundle By Name(w958) -> ("Disable plot"=w959:bool)
        n429 = case shown="False" w959 {
          tunnel: w958 -> [w970 _]
          frame False {
            # "Plot loop"
            n430 = Unbundle By Name(w970) -> ("Sweep buffer"=w973:dbl[][], "Readout buffer"=w972:dbl[][], "Xparameter"=w962:dbl, "Channel"=w968:dbl)
            n431 = local read "Exp_params"() -> (w969:T15)
            n432 = Equal?(x=w962, y=0.0) -> (x = y?=w967:bool)
            n433 = Decrement(x=w962) -> (x-1=w963:dbl)
            n434 = case shown="True" w967 {
              tunnel: w969 -> [w986 w995]
              tunnel: w968 -> [w985 w994]
              tunnel: w963 -> [w976 w989]
              tunnel: [w975 "counter"] -> w964
              tunnel: [w974 w988] -> w965
              frame False {
                n435 = call "Plot_build_legend.vi"("Y_id"=w985, "X_id"=w976, "Exp_params"=w986) -> ("Yunit"=w977:string, "Yname"=w978:string, "Xunit"=w979:string, "Xname"=w982:string)  [unwired: 3 in]
                n436 = Concatenate Strings(w978, " (", w977, ")") -> (w974:string)
                n437 = Concatenate Strings(w982, " (", w979, ")") -> (w975:string)
              }
              frame True {
                n438 = call "Plot_build_legend.vi"("Y_id"=w994, "X_id"=w989, "Exp_params"=w995) -> ("Yunit"=w990:string, "Yname"=w991:string)  [unwired: 3 in, 2 out]
                n439 = Concatenate Strings(w991, " (", w990, ")") -> (w988:string)
              }
            }
            n440 = Index Array(array=w972, index (col)=w968) -> (element=w960:dbl[])  [unwired: 1 in]
            n441 = Index Array(array=w973, index (col)=w962) -> (element=w961:dbl[])  [unwired: 1 in]
            n442 = Bundle("Sweep buffer"=w961, "Readout buffer"=w960) -> (→"Graph":T1)  [unwired: 1 in]
            n443 = property on="Graph" class="XYGraph (strict)"("YScale.NameLbl.Text"=w965) -> ()  [unwired: 2 in, 2 out]
            n444 = property on="Graph" class="XYGraph (strict)"("XScale.NameLbl.Text"=w964) -> ()  [unwired: 2 in, 2 out]
          }
          frame True {
          }
        }
      }
      frame #2 {
        n445 = local read "Timings"() -> (w999:dbl[][])
        n446 = Tick Count (ms)() -> (millisecond timer value=w996:u32)
        n447 = call "Timer.vi"("index"=2, "Timings in"=w999, "t1"=w1000, "t2"=w996) -> ("Timings out"=w998:dbl[][])  [unwired: 2 in]
        n448 = local write "Timings"(w998) -> ()
      }
    }
    n449 = local read "Finish"() -> (w956:bool)
  }
